vi "УОПП ПользователиZZ.vi"() -> ()   [LabVIEW 2018]
uses:
  Control 1.ctl
  <vilib>/Analysis/baseanly.llb/Mean (DBL).vi
  <vilib>/Instr/_visa.llb/VISA Configure Serial Port (Instr).vi
  <vilib>/Utility/file.llb/Write Delimited Spreadsheet (string).vi
  <vilib>/addons/control/pid/pid.llb/PID (DBL).vi
  <vilib>/NI/Modbus Library/API/Master/Modbus Master.lvclass
  <vilib>/addons/control/pid/NI_PID_pid.lvlib
  <vilib>/Analysis/NI_AALBase.lvlib
  <vilib>/Analysis/NI_AALPro.lvlib
panel:
  out "x > y?":bool
  in  "Наименование образца":string
  in  "OK Button 2":bool
  in  "OK Button":bool
  in  "Масса. г":dbl format="%#.3g"
  in  "Длина, мм.":dbl=30.0 min=8.0 max=150.0
  in  "Диаметр, мм.":dbl=30.0 min=8.0 max=100.0
  in  "клапан":u16=4000 format="%.3f"
  out "Boolean 10":bool
  out "Скорость падения давления":dbl format="%#.6g"
  out "y":dbl
  out "Вр1 2":dbl
  out "Вр2 3":dbl
  out "травление":bool
  out "травление3":bool
  out "травление 2":bool
  in  "error out":errorcluster
  out "Вр2":bool
  out "Boolean 9":bool
  out "Вр1":bool
  out "Boolean 7":bool
  out "Boolean 6":bool
  out "Boolean 5":bool
  out "Boolean 4":bool
  out "Boolean 3":bool
  in  "Штангель":dbl format="%#.3g"
  out "Время":dbl[](array[numeric])
  out "Пересчет":dbl[](array[numeric])
  out "Atm":dbl[](array[numeric])
  out "Vip":dbl[](array[numeric])
  out "Вип":dbl
  out "Вип 3":dbl
  out "Вип 2":dbl
  out "Вип 4":dbl
  out "Вип 5":dbl
  out "pori 4":dbl
  out "pori 2":dbl
  out "Tab Control 2":enum32{"Page 1", "Page 2", "Page 3"}(tab)=enum."Page 3"
  out "Проницаемость. мД":dbl
  out "Пористость. %":dbl format="%#.6f"
  out "P_пл.МПа":dbl format="%#.2g"
  out "P пл. МПа":dbl format="%#.2g"
  out "P гор. МПа":dbl format="%#.2g"
  out "Нижний":bool
  out "Верхний":bool
  out "K11":bool
  out "K10":bool
  out "K9":bool=TRUE
  out "K8":bool
  out "K7":bool
  out "K6":bool
  out "K5":bool
  out "K4":bool
  out "K3":bool
  out "K2":bool
  out "K1":bool
  out "Плотность образца.\n г/см3":dbl format="%#.3g"
  out "Объем скелета . см3":dbl format="%#.3g"
  out "Плотность зерен г/см3":dbl format="%#.3g"
  out "Плотность зерен г/см3":dbl
  out "Скорость":dbl format="%#.3g"
  out "Температура":dbl format="%#.3f"
  out "Пласт1":dbl format="%#.3g"
  out "Пласт2":dbl format="%#.3g"
  out "Ошибки":i32=1 format="%.3f"
  out "дельта":dbl format="%#.3g"
  in  "Регулятор\n давления":dbl min=0.0 max=1.5 format="%#.3f"
  in  "Пластовое давл.":dbl=1.5 min=0.0 max=1.5 format="%#.3g"
  out "Рпласт.":dbl(graph)
  in  "Min":dbl=0.05 format="%#.3g"
  in  "Max":dbl=0.62 format="%#.3g"
  out "Y":dbl format="%#.3g"
  out "X":dbl format="%#.3g"
  out "Pатм. МПа":dbl format="%#.3f"
  out "Пористость. %":dbl format="%#.3f"
  out "P2/P1":dbl[](array[numeric])
  out "Pпластовое":dbl format="%#.5f"
  out "Проницаемость. мД":dbl format="%#.3g"
  out "P_пластовое МПа":dbl format="%#.6f"
  out "Объем скелета . см3":dbl format="%#.3g"
  out "Плотность образца.\n г/см3":dbl format="%#.3g"
  out "0,17":dbl
  out "0,2":dbl
  out "0,25":dbl
  out "0,15":dbl
  out "D 0,4":dbl
  in  "stop 3":bool=TRUE
  in  "Клапана":bool[](array[boolean])=[FALSE, FALSE, FALSE, FALSE, FALSE, FALSE, FALSE, FALSE, TRUE, FALSE, FALSE, FALSE, FALSE]
  out "String 2":T1="     К1         К2         К3         К4          К5          К6         К7         К8         К9        К10         К11 "
  in  "Продувка":bool
  out "n 1":dbl
  out "n 2":dbl
  out "n 3":dbl
  out "n 4":dbl
  out "n":dbl
  out "D2":dbl
  out "D3":dbl
  out "D4":dbl
  out "D1":dbl
  out "Q":dbl
  out "Q 2":dbl
  out "Q 3":dbl
  out "Q 4":dbl
  out "Q 3.2":dbl
  out "pori 3":dbl
  out "XY Graph 2":cluster{dbl[], dbl[]}[](graph)
  out "секунды 2":dbl format="%#.3g"
  out "0,38":dbl
  out "Low level pronic":dbl
  out "pori 1":dbl
  out "T0.5":u32
  out "T1":u32
  out "T2":u32
  out "appended array":dbl[](array[numeric])
  out "sum":dbl
  out "Прол":dbl
  in  "Сохранение данных":bool
  in  "Укажите место для сохранения файла":path
  in  "Boolean 8":bool
  out "Table Control":string[][](table)
  in  "Save Button":bool=TRUE
  in  "stop 2":bool
  in  "Режимы":u16(ring)=1 items=["Проницаемость", "Пористость"]
  in  "Старт":bool
  out "Темп":dbl format="%0.2f"
  in  "Up Button":bool
  in  "Down Button":bool
  out "Р горное, МПа":sgl format="%#.2f"
  in  "Мультипликатор":dbl(slide) min=0.0 max=70.0 scale=0.0..70.0
  out "Атмосферное":dbl(knob) scale=0.0..1.0
  in  "код":string
  in  "Калибровка":bool
  in  "РД-1 1,0 МПА":dbl min=0.0 max=100.0 step=0.01 format="%#.3f"
  in  "РД-2 1,0 МПА":dbl=0.078 min=0.0 max=100.0 step=0.01 format="%#.2f"
  in  "PID gains":T2={"proportional gain (Kc)"=50.0, "integral time (Ti, min)"=4.0, "derivative time (Td, min)"=0.0} {"derivative time (Td, min)" format="%.3f"; "integral time (Ti, min)" format="%.3f"; "proportional gain (Kc)" format="%.3f"}
  out "output":dbl=4000.0 format="%.2f"
  in  "dt (s)":dbl=5.0 format="%.3f"
  in  "baud rate (9600)":u32=9600
  in  "ms to wait":u32=40
  out "Press":dbl format="%5.6f"
  out "Boolean 2":bool=TRUE
  out "Numeric 2":i32
  out "Numeric":i32
  # "Введите параметры образца"
  # "К 30"
  # "К 100"
  # "N2"
  # "Регулятор\n давления"
  # "He"
  # "Емкость 1"
  # "Емкость 2"
  # "Емкость 3"
  # "Емкость 4"
  # "Емкость 5"
  # "Емкость 6"
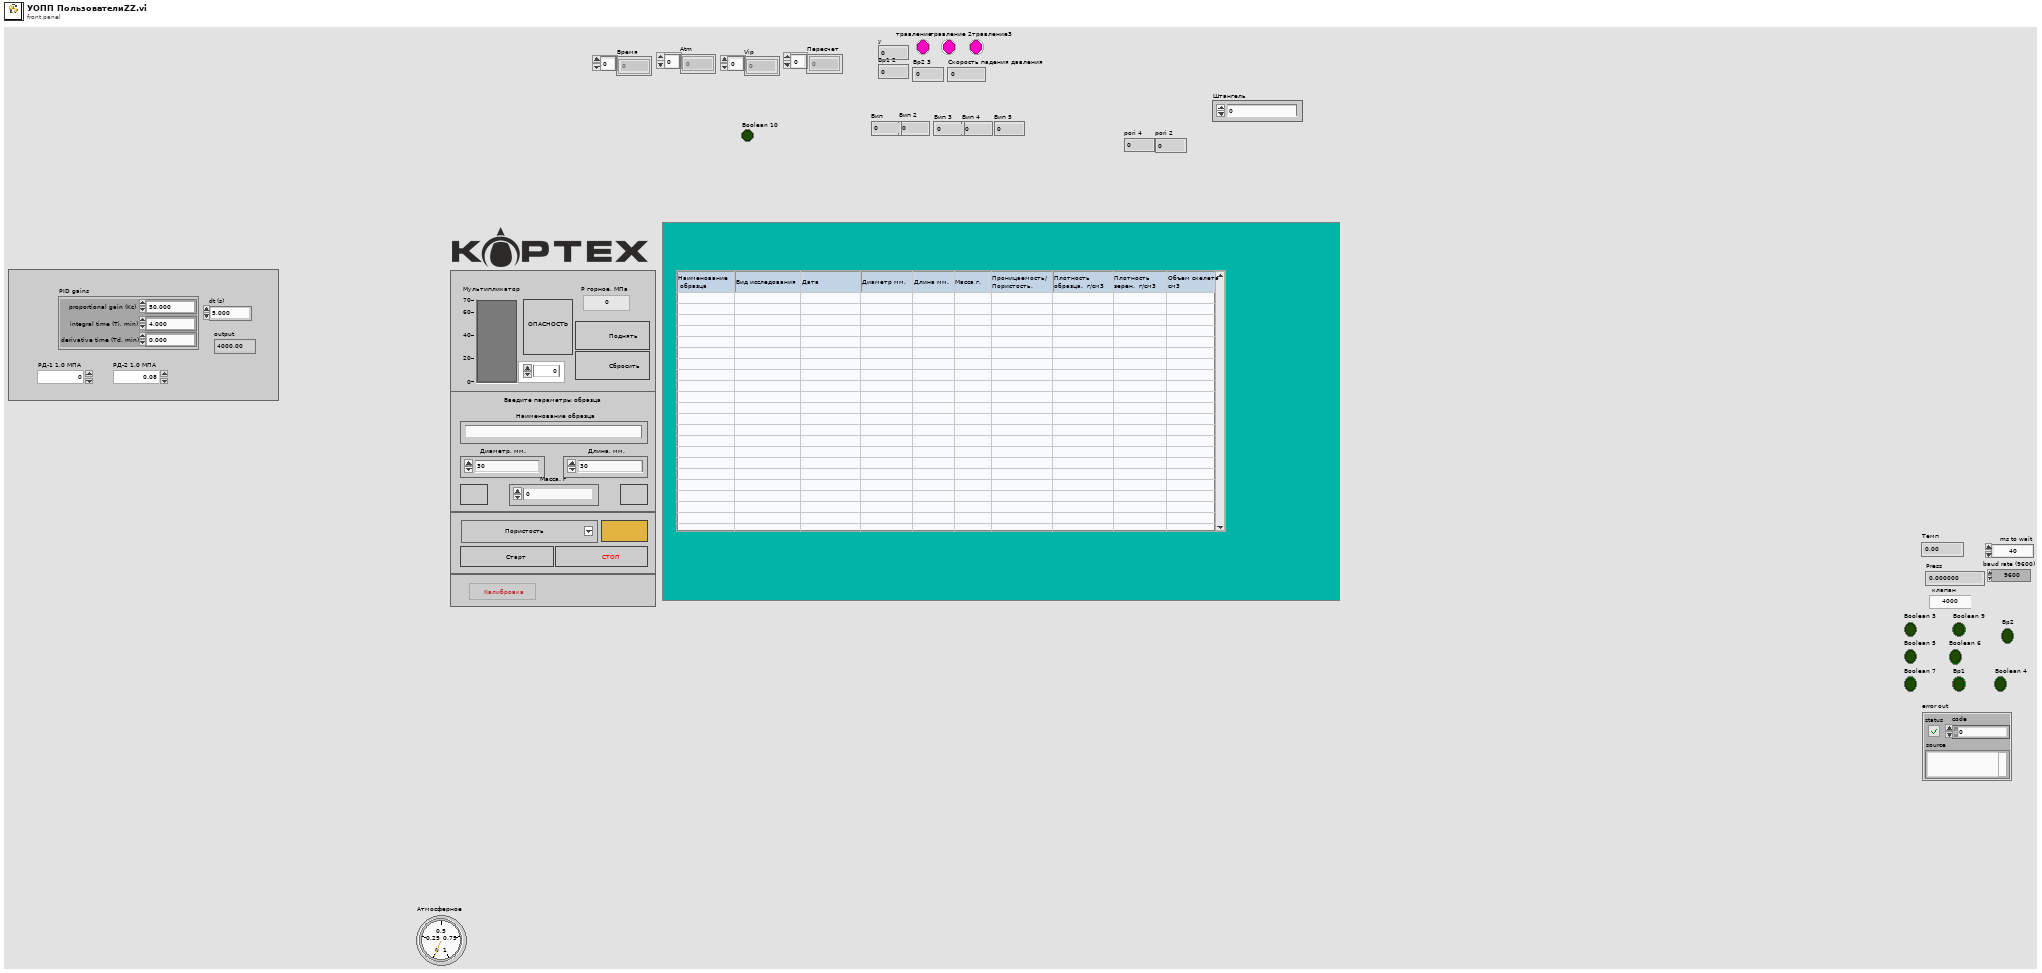
[diagram p1: front panel]
types:
  T1 = typedef "Control 1.ctl" = string
  T2 = cluster{"proportional gain (Kc)":dbl, "integral time (Ti, min)":dbl, "derivative time (Td, min)":dbl}
  T3 = enum8{"Enabled", "Disabled", "Disabled and Grayed Out"}
  T4 = typedef "Датчики.ctl" = cluster{"Клапана":T5, "Концевики":T6, "Рег.давления":T7, "Давления":cluster{"Р горное":sgl, "Р пластовое":sgl, "Р атм.":sgl, "Температура":sgl, "Р_пластовое":sgl}}
  T5 = typedef "Клапана.ctl" = cluster{"Ka-1":bool, "Ka-2":bool, "Ka-3":bool, "Ka-4":bool, "Ka-5":bool, "Ka-6":bool, "Ka-7":bool, "Ka-8":bool, "Ka-9":bool, "Ka-10":bool, "Ka-11":bool, "Ka-12":bool, "Ka-13":bool}
  T6 = typedef "Концевики.ctl" = cluster{"Di-1":bool, "Di-2":bool}
  T7 = typedef "Регуляторы.ctl" = cluster{"Рег.№1":u16, "Рег.№2":u16, "Рег.№3":u16}
  T8 = cluster{"Время":dbl[], "Best Polynomial Fit":dbl[]}
  T9 = cluster{"Время":dbl[], "Best Polynomial Fit":dbl[]}[]
  T10 = enum32{"invalid app kind", "Development System", "Run Time System", "Student Edition", "Embedded LabVIEW", "Evaluation", "Custom"}
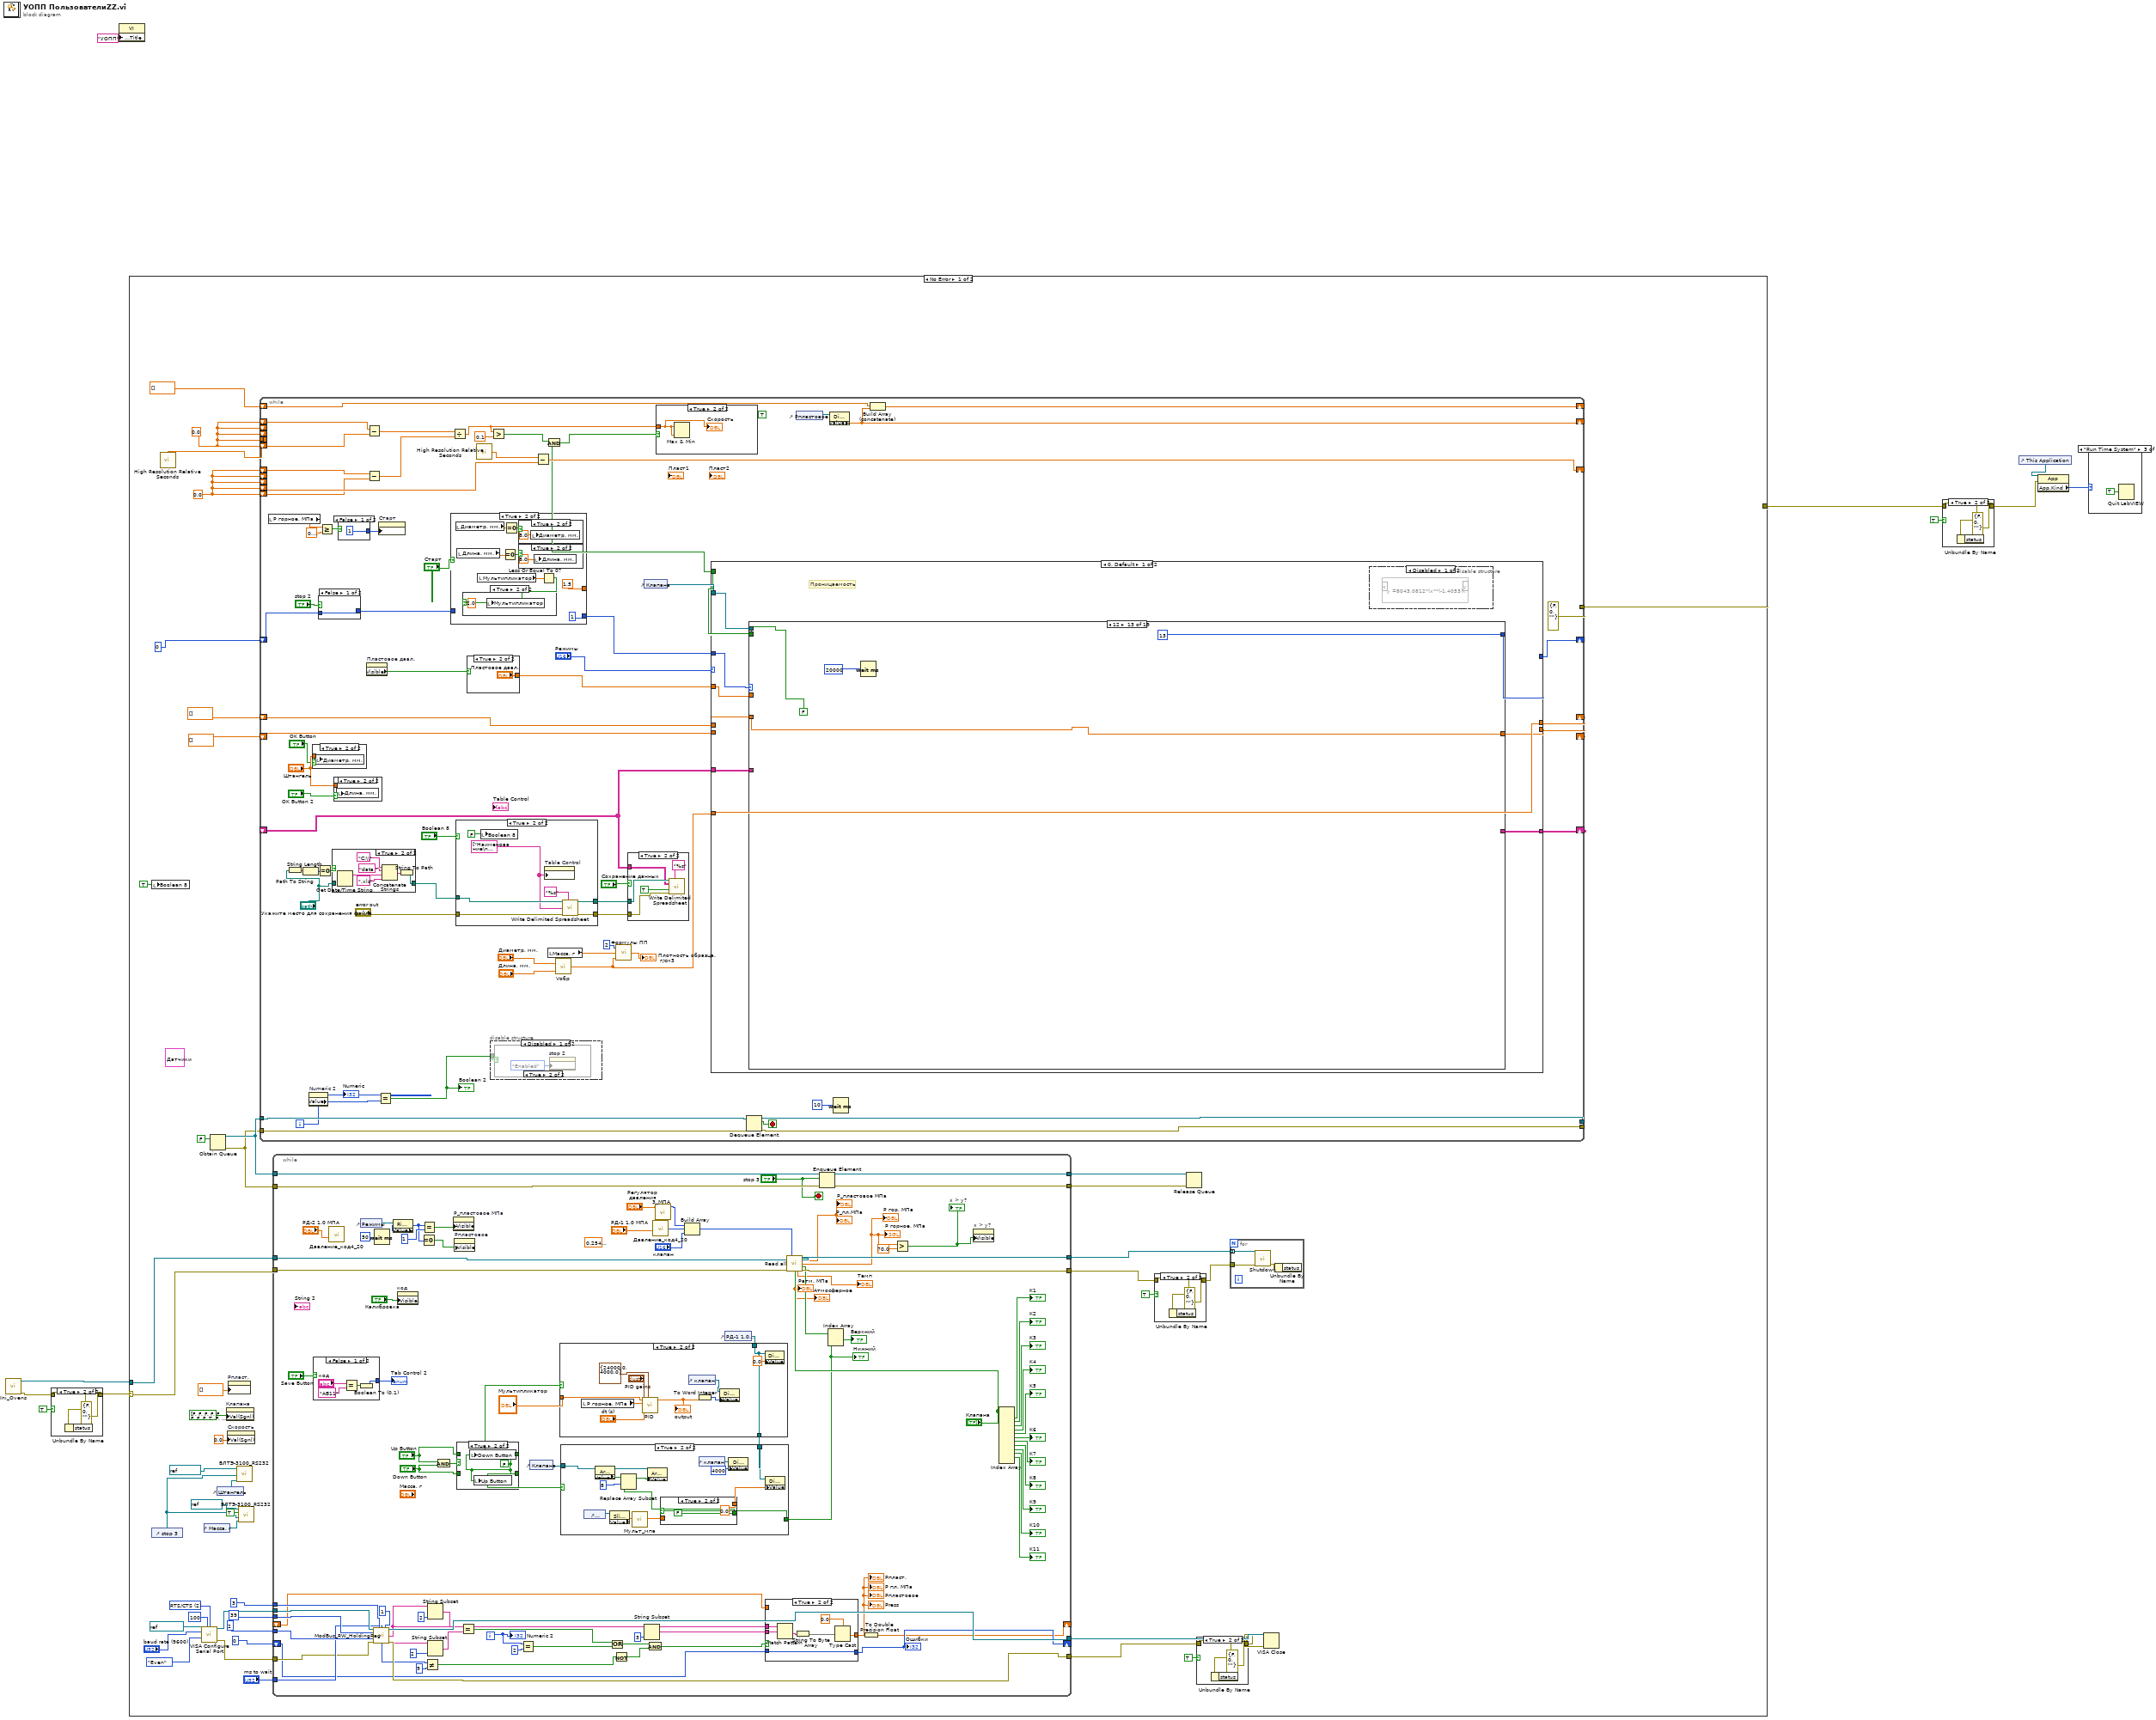
[diagram p0: block diagram]
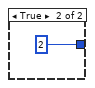
[diagram p8: hidden frame]
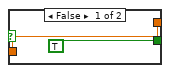
[diagram p11: hidden frame]
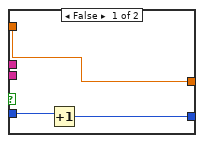
[diagram p12: hidden frame]
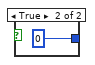
[diagram p15: hidden frame]
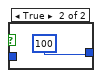
[diagram p18: hidden frame]
diagram:
  n1 = call "Ini_Ovens.vi"() -> ("error out"=w5:errorcluster, "Овны"=w10:refnum<class "Modbus Master.lvclass">[])  [unwired: 10 in]
  n2 = case shown="True" TRUE {
    tunnel: [w11 errorcluster {"status"=FALSE, "code"=0, "source"=""} ("error IO")] -> w6
    tunnel: w5 -> [w11 w12]
    frame False {
    }
    frame True {
      n3 = Unbundle By Name(w12) -> ()  [unwired: 1 out]
    }
  }
  n4 = property class="VI"("Front Panel Window:Title"="УОПП") -> ()  [unwired: 2 in, 2 out]
  n5 = case shown="No Error" w6 {
    selector: w6 -> [w51 _]
    tunnel: w10 -> [w50 _]
    tunnel: [w49 _] -> w3
    frame No Error {
      w36 = u16 2 items=["None", "XON/XOFF", "RTS/CTS", "XON/XOFF & RTS/CTS", "DTR/DSR", "XON/XOFF & DTR/DSR"] ("flow control (0:none)")
      w43 = 0.0
      w48 = 0.0
      (unwired) T4 {"Клапана"={"Ka-1"=FALSE, "Ka-2"=FALSE, "Ka-3"=FALSE, "Ka-4"=FALSE, "Ka-5"=FALSE, "Ka-6"=FALSE, "Ka-7"=FALSE, "Ka-8"=FALSE, "Ka-9"=FALSE, "Ka-10"=FALSE, "Ka-11"=FALSE, "Ka-12"=FALSE, "Ka-13"=FALSE}, "Концевики"={"Di-1"=FALSE, "Di-2"=FALSE}, "Рег.давления"={"Рег.№1"=0, "Рег.№2"=0, "Рег.№3"=0}, "Давления"={"Р горное"=0.0, "Р пластовое"=0.0, "Р атм."=0.0, "Температура"=0.0, "Р_пластовое"=0.0}} ("Датчики")
      n6 = local write "Boolean 8"(TRUE ("Boolean 8")) -> ()
      n7 = control-ref of="stop 3"() -> (w14:refnum<vi>)
      n8 = call <vilib>:"High Resolution Relative Seconds.vi"() -> ("relative seconds"=w47:dbl)
      n9 = call-poly "VISA Configure Serial Port"("VISA resource name"=refnum<visa-resource-name> "COM10" ("VISA Refnum in"), "timeout (10sec)"=u32 100, "baud rate (9600)"="baud rate (9600)", "parity (0:none)"=enum16{"None", "Odd", "Even", "Mark", "Space"}."Even", "flow control (0:none)"=w36) -> ("VISA resource name out"=w33:refnum<visa-resource-name>, "error out"=w31:errorcluster)  [unwired: 9 in]
      n10 = control-ref of="Масса. г"() -> (w19:refnum<vi>)
      n11 = Obtain Queue(element data type=FALSE) -> (queue out=w57:refnum<queue>, error out=w44:errorcluster)  [unwired: 4 in, 1 out]
      n12 = control-ref of="Штангель"() -> (w15:refnum<vi>)
      n13 = property on="Клапана" class="Arr (strict)"("Val(Sgnl)"=bool[] [FALSE, FALSE, FALSE, FALSE, FALSE, FALSE, FALSE, FALSE, TRUE, FALSE, FALSE, FALSE, FALSE] ("Value (Signaling)")) -> ()  [unwired: 2 in, 2 out]
      n14 = property on="Скорость" class="DigNum (strict)"("Val(Sgnl)"=0.0 ("Value (Signaling)")) -> ()  [unwired: 2 in, 2 out]
      n15 = property on="Рпласт." class="WFChart (strict)"("History Data"=sgl[] []) -> ()  [unwired: 2 in, 2 out]
      n16 = call "ВЛТЭ-3100_RS232.vi"("Balance 2"=w15, "Stop 2"=w14, "VISA resource name"=refnum<visa-resource-name> "COM3") -> ()  [unwired: 2 in]
      n17 = call "ВЛТЭ-3100_RS232.vi"("Balance 2"=w19, "Stop 2"=w14, "0,001"=TRUE, "VISA resource name"=refnum<visa-resource-name> "COM5") -> ()  [unwired: 1 in]
      n18 = while {
        tunnel: w57 -> [w268]
        tunnel: w44 -> [w266]
        tunnel: [w265] -> _
        tunnel: [w264] -> _
        tunnel: [errorcluster {"status"=FALSE, "code"=0, "source"=""} ("error in (no error)")] -> w49
        shift-right: [w245] -> _
        shift-left: w48 -> [w261]
        shift-left: w48 -> [_]
        shift-left: w48 -> [_]
        shift-left: w48 -> [_]
        shift-left: w48 -> [w260]
        shift-right: [w257] -> _
        shift-left: w43 -> [w256]
        shift-left: w43 -> [_]
        shift-left: w43 -> [_]
        shift-left: w43 -> [_]
        shift-left: w43 -> [w255]
        tunnel: w47 -> [w258]
        shift-right: [w247] -> _
        shift-left: 0 -> [w223]
        shift-right: [w237] -> _
        shift-left: dbl[] [] -> [w238]
        shift-right: [w234] -> _
        shift-left: dbl[] [] -> [w233]
        shift-right: [w231] -> _
        shift-left: dbl[] [] -> [w232]
        shift-right: [w207] -> _
        shift-left: _ -> [w206]
        i -> [w241]
        stop <- w267 stop-if-true
        (unwired) TRUE
        n19 = local read "Р горное, МПа"() -> (w221:sgl)
        n20 = Path To String(path="Укажите место для сохранения файла") -> (string=w214:string)
        n21 = String Length(string=w214) -> (length=w215:i32)
        n22 = property on="Numeric 2" class="DigNum (strict)"() -> ("Value"=w243:i32)  [unwired: 2 in, 2 out]
        n23 = case shown="True" "OK Button" {
          tunnel: "Штангель" -> [_ w295]
          frame False {
          }
          frame True {
            n24 = local write "Диаметр, мм."(w295) -> ()
          }
        }
        n25 = Equal To 0?(x=w215) -> (x = 0?=w213:bool)
        n26 = case shown="False" "stop 2" {
          tunnel: w223 -> [w292 _]
          tunnel: [w292 100] -> w222
          frame False {
          }
          frame True {
          }
        }
        n27 = Greater Or Equal?(x=w221, y=sgl 0.9) -> (x >= y?=w218:bool)
        n28 = case shown="True" w213 {
          tunnel: "Укажите место для сохранения файла" -> [w276 _]
          tunnel: [w276 w277] -> w211
          frame False {
          }
          frame True {
            n29 = Get Date/Time String() -> (date string=w282:string)  [unwired: 3 in, 1 out]
            n30 = Concatenate Strings("C:\\" ("string"), "data " ("default name"), w282, ".xls" ("string")) -> (w278:string)
            n31 = String To Path(string=w278) -> (path=w277:path)
          }
        }
        n32 = case shown="True" "OK Button 2" {
          tunnel: "Штангель" -> [_ w294]
          frame False {
          }
          frame True {
            n33 = local write "Длина, мм."(w294) -> ()
          }
        }
        n34 = case shown="False" w218 {
          tunnel: [1 0] -> w219
          frame False {
          }
          frame True {
          }
        }
        n35 = Subtract(x=w261, y=w260) -> (x-y=w254:dbl)
        n36 = Subtract(x=w256, y=w255) -> (x-y=w253:dbl)
        n37 = property on="Пластовое давл." class="DigNum (strict)"() -> ("Visible"=w235:bool)  [unwired: 2 in, 2 out]
        n38 = Equal?(x=w241, y=w243) -> (x = y?=w242:bool)
        "Boolean 2" <- w242
        n39 = property on="Старт" class="Bool (strict)"("DisabledEnum"=w219) -> ()  [unwired: 2 in, 2 out]
        n40 = case shown="True" "Старт" {
          tunnel: [w1028 1] -> w246
          tunnel: [0.0 ("Начальное давл.") 1.5 ("Начальное давл.")] -> _
          tunnel: w222 -> [w1028 _]
          frame False {
          }
          frame True {
            n41 = local read "Диаметр, мм."() -> (w1033:dbl)
            n42 = local read "Длина, мм."() -> (w1031:dbl)
            n43 = local read "Мультипликатор"() -> (w1034:dbl)
            n44 = Equal To 0?(x=w1031) -> (x = 0?=w1030:bool)
            n45 = Equal To 0?(x=w1033) -> (x = 0?=w1032:bool)
            n46 = case shown="True" w1032 {
              frame False {
              }
              frame True {
                n47 = local write "Диаметр, мм."(8.0 ("Диаметр. мм.")) -> ()
              }
            }
            n48 = case shown="True" w1030 {
              frame False {
              }
              frame True {
                n49 = local write "Длина, мм."(8.0 ("Диаметр. мм.")) -> ()
              }
            }
            n50 = Less Or Equal To 0?(x=w1034) -> (x <= 0?=w1035:bool)
            n51 = case shown="True" w1035 {
              frame False {
              }
              frame True {
                n52 = local write "Мультипликатор"(2.0 ("Мультиплексор.МПА")) -> ()
              }
            }
          }
        }
        n53 = Divide(x=w254, y=w253) -> (x/y=w252:dbl)
        n54 = case shown="True" "Boolean 8" {
          tunnel: [w284 w290] -> w209
          tunnel: [w283 w289] -> w208
          tunnel: w211 -> [w284 w286]
          tunnel: "error out" -> [w283 w288]
          frame False {
          }
          frame True {
            w285 = string[] ["Наименование\n образца", "Вид исследования", "Дата", "Диаметр мм.", "Длина мм.", "Масса г.", "Проницаемость/\nПористость.", "Плотность\nобразца.  г/см3", "Плотность\nзерен.  г/см3", "Объем скелета\nсм3 "] ("Array 2")
            n55 = local write "Boolean 8"(FALSE ("Boolean 8")) -> ()
            n56 = property on="Table Control" class="Tbl (strict)"("Column Headers[]"=w285) -> ()  [unwired: 2 in, 2 out]
            n57 = call-poly <vilib>:"Write Delimited Spreadsheet.vi"("file path (dialog if empty)"=w286, "format (%s)"="%s", "1D data"=w285, "error in (no error)"=w288) -> ("new file path (Not A Path if cancelled)"=w290:path, "error out"=w289:errorcluster)  [unwired: 10 in]
          }
        }
        n58 = case shown="True" w235 {
          tunnel: [1.5 ("Пластовое давл.") "Пластовое давл."] -> w239
          frame False {
          }
          frame True {
          }
        }
        n59 = call <vilib>:"High Resolution Relative Seconds.vi"() -> ("relative seconds"=w259:dbl)
        n60 = disable-structure shown="Disabled" {
          disable-tunnel: w242 -> [w296 _]
          frame Disabled {
            n61 = case shown="True" w296 {
              frame False {
              }
              frame True {
                n62 = property on="stop 2" class="Bool (strict)"("DisabledEnum"=T3."Enabled" ("Disabled")) -> ()  [unwired: 2 in, 2 out]
              }
            }
          }
          frame Enabled {
          }
        }
        n63 = Greater?(x=w252, y=0.1) -> (0:w250:bool)
        n64 = Subtract(x=w259, y=w258) -> (x-y=w257:dbl)
        n65 = local read "Масса. г"() -> (w204:dbl)
        n66 = call "Vобр.vi"("Длина, мм."="Длина, мм.", "Диаметр. мм."="Диаметр, мм.") -> ("Объем образца см3"=w203:dbl)
        n67 = call "Формулы ПП.vi"("PerB"=w203, "PerA"=w204, "mode"=2) -> ("Exid"=→"Плотность образца.\n г/см3":dbl)
        n68 = case shown="True" "Сохранение данных" {
          tunnel: w209 -> [_ w271]
          tunnel: w208 -> [_ w270]
          tunnel: w206 -> [_ w269]
          frame False {
          }
          frame True {
            n69 = call-poly <vilib>:"Write Delimited Spreadsheet.vi"("file path (dialog if empty)"=w271, "format (%s)"="%s" ("format (%.3f)"), "2D data"=w269, "append to file? (new file:F)"=TRUE, "error in (no error)"=w270) -> ()  [unwired: 9 in, 2 out]
          }
        }
        n70 = control-ref of="Клапана"() -> (w248:refnum<vi>)
        n71 = case shown="0, Default" "Режимы" {
          tunnel: w248 -> [w308 w737]
          tunnel: [w302 w734] -> w247
          tunnel: w246 -> [w306 w735]
          tunnel: [w307 w733] -> w244
          tunnel: w239 -> [w309 w736]
          tunnel: [w305 w732] -> w234
          tunnel: w233 -> [w305 w731]
          tunnel: w232 -> [w304 w730]
          tunnel: [w303 w730] -> w231
          tunnel: w203 -> [_ w729]
          tunnel: [w300 w728] -> w207
          tunnel: w206 -> [w301 w727]
          frame 0, Default {
            # "Проницаемость"
            n72 = case shown="12" w306 {
              selector: w306 -> [w314 _ _ _ _ _ _ _ _ _ _ _ _ _ _ _ _ _ _]
              tunnel: [w314 2 w333 4 5 6 7 w416 9 10 11 12 13 14 0 51 52 7 w691] -> w302
              tunnel: w308 -> [_ w325 _ w357 _ w378 _ _ _ _ _ w618 _ w634 _ w647 _ w681 w694]
              tunnel: [FALSE FALSE FALSE FALSE FALSE FALSE FALSE FALSE FALSE FALSE FALSE TRUE FALSE FALSE FALSE FALSE FALSE FALSE FALSE] -> w307
              tunnel: w309 -> [_ w321 _ _ _ _ _ _ _ _ _ _ _ _ _ _ _ _ _]
              tunnel: w304 -> [w311 w319 w336 w355 w366 w375 w386 _ w567 w590 w603 w614 w625 w631 w644 w655 w658 w683 w692]
              tunnel: [w310 w318 w335 w354 w365 w374 w385 w408 w566 dbl[] [] w602 w614 w625 w631 w644 w655 w658 w683 w692] -> w303
              tunnel: [_ _ _ _ _ _ _ _ _ _ w600 _ _ _ _ _ _ _ _] -> w300
              tunnel: w301 -> [_ _ _ _ _ _ _ _ _ _ w598 _ _ _ _ _ _ _ _]
              frame 0, Default {
                n73 = local read "Темп"() -> (w312:dbl)
                n74 = Build Array (concatenate)(w311, w312) -> (w310:dbl[])
              }
              frame 1 {
                w315 = 0.0 ("Пористость. %")
                w316 = TRUE ("new element/subarray")
                n75 = property on="Регулятор\n давления" class="DigNum (strict)"("Value"=w321) -> ()  [unwired: 2 in, 2 out]
                n76 = property class="Arr (strict)"(reference=w325) -> (reference out=w328:refnum<vi>, error out=w327:errorcluster, "Value"=w329:bool[])  [unwired: 1 in]
                n77 = Replace Array Subset(array=w329, new element #1=w316, index #1=0 ("index"), new element #2=w316, index #2=9 ("index"), new element #3=w316, index #3=4, new element #4=w316, index #4=2 ("index"), new element #5=w316, index #5=5 ("index")) -> (w326:bool[])
                n78 = property class="Arr (strict)"(reference=w328, error in=w327, "Value"=w326) -> ()  [unwired: 2 out]
                n79 = local read "Темп"() -> (w320:dbl)
                n80 = Build Array (concatenate)(w319, w320) -> (w318:dbl[])
                n81 = local write "Пористость. %"(w315) -> ()
                n82 = local write "Плотность образца.\n г/см3"(w315) -> ()
                n83 = local write "Объем скелета . см3"(w315) -> ()
                n84 = local write "Плотность зерен г/см3"(w315) -> ()
                n85 = local write "Проницаемость. мД"(w315) -> ()
              }
              frame 2 {
                n86 = call <vilib>:"High Resolution Relative Seconds.vi"() -> ("relative seconds"=w334:dbl)
                n87 = while {
                  tunnel: w334 -> [w347]
                  tunnel: [3] -> w333
                  stop <- w340 stop-if-true
                  n88 = local read "Max"() -> (w339:dbl)
                  n89 = call <vilib>:"High Resolution Relative Seconds.vi"() -> ("relative seconds"=w348:dbl)
                  n90 = Subtract(x=w348, y=w347) -> (x-y=w346:dbl)
                  n91 = property on="Pпластовое" class="DigNum (strict)"() -> ("Value"=w349:dbl)  [unwired: 2 in, 2 out]
                  n92 = Greater Or Equal?(x=w346, y=120.0) -> (x >= y?=w342:bool)
                  n93 = Greater?(x=w349, y=w339) -> (0:w343:bool)
                  n94 = local read "stop 2"() -> (w341:bool)
                  n95 = Compound Arithmetic op=OR(w343, w342, w341) -> (w340:bool)
                }
                n96 = local read "Темп"() -> (w337:dbl)
                n97 = Build Array (concatenate)(w336, w337) -> (w335:dbl[])
              }
              frame 3 {
                w352 = FALSE ("new element/subarray")
                (unwired) 1.5 ("VPPL-3L")
                n98 = property on="Регулятор\n давления" class="DigNum (strict)"("Value"=0.0 ("VPPL-3L")) -> ()  [unwired: 2 in, 2 out]
                n99 = property class="Arr (strict)"(reference=w357) -> (reference out=w360:refnum<vi>, error out=w361:errorcluster, "Value"=w359:bool[])  [unwired: 1 in]
                n100 = property on="Регулятор\n давления" class="DigNum (strict)"("Value"=0.0 ("VPPL-3L")) -> ()  [unwired: 2 in, 2 out]
                n101 = Replace Array Subset(array=w359, new element #1=w352, index #1=0 ("index"), new element #2=w352, index #2=9 ("index")) -> (w362:bool[])
                n102 = property class="Arr (strict)"(reference=w360, error in=w361, "Value"=w362) -> ()  [unwired: 2 out]
                n103 = local read "Темп"() -> (w356:dbl)
                n104 = Build Array (concatenate)(w355, w356) -> (w354:dbl[])
              }
              frame 4 {
                n105 = Wait (ms)(milliseconds to wait=u32 15000) -> ()  [unwired: 1 out]
                n106 = local read "Темп"() -> (w367:dbl)
                n107 = Build Array (concatenate)(w366, w367) -> (w365:dbl[])
              }
              frame 5 {
                w371 = TRUE ("Boolean 3")
                n108 = local write "травление"(w371) -> ()
                n109 = local write "травление 2"(w371) -> ()
                n110 = local write "травление3"(w371) -> ()
                n111 = local write "Boolean 9"(w371) -> ()
                n112 = property class="Arr (strict)"(reference=w378) -> (reference out=w372:refnum<vi>, error out=w382:errorcluster, "Value"=w383:bool[])  [unwired: 1 in]
                n113 = Replace Array Subset(array=w383, new element=TRUE ("new element/subarray"), index=3) -> (w381:bool[])
                n114 = property class="Arr (strict)"(reference=w372, error in=w382, "Value"=w381) -> ()  [unwired: 2 out]
                n115 = local read "Темп"() -> (w376:dbl)
                n116 = Build Array (concatenate)(w375, w376) -> (w374:dbl[])
                "Boolean 3" <- w371
                "Boolean 4" <- w371
                "Boolean 5" <- w371
                "Boolean 6" <- w371
                "Boolean 7" <- w371
              }
              frame 6 {
                n117 = call <vilib>:"High Resolution Relative Seconds.vi"() -> ("relative seconds"=w388:dbl)
                n118 = while {
                  tunnel: [w401] -> _
                  shift-right: [w397] -> w385
                  shift-left: w386 -> [w398]
                  tunnel: w388 -> [w395]
                  stop <- w392 stop-if-true
                  (unwired) 1600000 ("x")
                  n119 = call <vilib>:"High Resolution Relative Seconds.vi"() -> ("relative seconds"=w396:dbl)
                  n120 = property on="Max" class="DigNum (strict)"() -> ("Visible"=w400:bool)  [unwired: 2 in, 2 out]
                  n121 = Subtract(x=w396, y=w395) -> (x-y=w394:dbl)
                  n122 = case shown="True" w400 {
                    tunnel: [0.7 "Max"] -> w401
                    frame False {
                    }
                    frame True {
                    }
                  }
                  n123 = property on="Pпластовое" class="DigNum (strict)"() -> ("Value"=w403:dbl)  [unwired: 2 in, 2 out]
                  n124 = Less Or Equal?(x=w403, y=w401) -> (x <= y?=w391:bool)
                  n125 = local read "stop 2"() -> (w389:bool)
                  n126 = Greater Or Equal?(x=w394, y=120.0) -> (x >= y?=w390:bool)
                  n127 = Wait Until Next ms Multiple(millisecond multiple=u32 10) -> ()  [unwired: 1 out]
                  n128 = Compound Arithmetic op=OR(w391, w390, w389) -> (w392:bool)
                  n129 = local read "Темп"() -> (w399:dbl)
                  n130 = Build Array (concatenate)(w398, w399) -> (w397:dbl[])
                }
              }
              frame 7 {
                w406 = TRUE ("Вр1")
                n131 = local write "Boolean 9"(w406) -> ()
                n132 = local write "Вр1"(w406) -> ()
                n133 = local write "Вр2"(w406) -> ()
                n134 = call <vilib>:"High Resolution Relative Seconds.vi"() -> ("relative seconds"=w413:dbl)
                n135 = while {
                  tunnel: [w446] -> w414 mode=indexing
                  tunnel: [w448] -> w409 mode=indexing
                  tunnel: w413 -> [w470]
                  tunnel: [w469] -> _
                  tunnel: [w422] -> w412 mode=indexing
                  shift-right: [w460] -> w408
                  shift-left: dbl[] [] -> [w467]
                  tunnel: [w461] -> w410 mode=indexing
                  stop <- w464 stop-if-true
                  (unwired) 2147483647 ("y")
                  n136 = property on="Min" class="DigNum (strict)"() -> ("Visible"=w468:bool)  [unwired: 2 in, 2 out]
                  n137 = local read "травление"() -> (w449:bool)
                  n138 = local read "травление 2"() -> (w450:bool)
                  n139 = local read "травление3"() -> (w451:bool)
                  n140 = case shown="True" w468 {
                    tunnel: [0.15 "Min"] -> w469
                    frame False {
                    }
                    frame True {
                    }
                  }
                  n141 = call <vilib>:"High Resolution Relative Seconds.vi"() -> ("relative seconds"=w471:dbl)
                  n142 = property on="Pпластовое" class="DigNum (strict)"() -> ("Value"=w448:dbl)  [unwired: 2 in, 2 out]
                  n143 = Subtract(x=w471, y=w470) -> (x-y=w446:dbl)
                  n144 = property on="Pатм. МПа" class="DigNum (strict)"() -> ("Value"=w461:dbl)  [unwired: 2 in, 2 out]
                  n145 = local read "Вр2"() -> (w452:bool)
                  n146 = local read "stop 2"() -> (w465:bool)
                  n147 = Greater Or Equal?(x=w446, y=20.0) -> (x >= y?=w453:bool)
                  n148 = local read "Вр1"() -> (w455:bool)
                  n149 = Greater Or Equal To 0?(x=w446) -> (x >= 0?=w456:bool)
                  n150 = And(x=w453, y=w452) -> (x .and. y?=w447:bool)
                  n151 = case shown="True" w447 {
                    selector: w447 -> [w477 _]
                    tunnel: [w477 w491] -> w438
                    tunnel: w451 -> [_ w480]
                    tunnel: w450 -> [_ w484]
                    tunnel: w449 -> [_ w486]
                    tunnel: w448 -> [_ w488]
                    frame False {
                    }
                    frame True {
                      n152 = local read "Вр1 2"() -> (w489:dbl)
                      n153 = Subtract(x=w488, y=w489) -> (x-y=w493:dbl)
                      n154 = Divide(x=w493, y=10.0) -> (x/y=w481:dbl)
                      "Скорость падения давления" <- w481
                      n155 = call "Больше И.vi"("Чек"=w480, "Граница"=0.0001 ("y"), "Значение"=w481) -> ("T/F"=w478:bool)
                      n156 = call "Больше И.vi"("Чек"=w486, "Граница"=0.00083 ("y"), "Значение"=w481) -> ("T/F"=w487:bool)
                      n157 = call "Больше И.vi"("Чек"=w484, "Граница"=0.00033 ("y"), "Значение"=w481) -> ("T/F"=w482:bool)
                      n158 = Compound Arithmetic op=OR(w487, w482, w478) -> (w491:bool)
                      "Вр2 3" <- w488
                      "Вр2" <- FALSE ("Вр2")
                    }
                  }
                  "Boolean 10" <- w438
                  n159 = Less Or Equal?(x=w448, y=w469) -> (x <= y?=w463:bool)
                  n160 = call "Формула Проницаемости.vi"("Р атм.."=w461, "P пластовое"=w448) -> ("Давление по пересчету"=w422:dbl)  [unwired: 9 in]
                  n161 = And(x=w456, y=w455) -> (x .and. y?=w454:bool)
                  n162 = Greater Or Equal?(x=w446, y=600.0) -> (x >= y?=w462:bool)
                  n163 = case shown="True" w454 {
                    tunnel: w448 -> [_ w495]
                    frame False {
                    }
                    frame True {
                      "Вр1 2" <- w495
                      "Вр1" <- FALSE ("Вр1")
                    }
                  }
                  n164 = local read "Темп"() -> (w459:dbl)
                  n165 = Build Array (concatenate)(w467, w459) -> (w460:dbl[])
                  n166 = call-poly <vilib>:"Mean.vi"("X"=w460) -> ("mean"=w458:dbl)  [unwired: 1 out]
                  n167 = local read "Boolean 9"() -> (w420:bool)
                  n168 = local read "Boolean 4"() -> (w433:bool)
                  n169 = local read "Boolean 3"() -> (w435:bool)
                  n170 = local read "Boolean 5"() -> (w429:bool)
                  n171 = local read "Boolean 6"() -> (w426:bool)
                  n172 = local read "Boolean 7"() -> (w424:bool)
                  n173 = call "Больше И.vi"("Чек"=w420, "Граница"=0.38 ("y"), "Значение"=w422) -> ("T/F"=w421:bool)
                  n174 = call "Больше И.vi"("Чек"=w429, "Граница"=0.2 ("y"), "Значение"=w422) -> ("T/F"=w431:bool)
                  n175 = call "Больше И.vi"("Чек"=w433, "Граница"=0.25 ("y"), "Значение"=w422) -> ("T/F"=w434:bool)
                  n176 = call "Больше И.vi"("Чек"=w435, "Граница"=0.4 ("y"), "Значение"=w422) -> ("T/F"=w437:bool)
                  n177 = call "Больше И.vi"("Чек"=w424, "Граница"=0.15 ("y"), "Значение"=w422) -> ("T/F"=w423:bool)
                  n178 = call "Больше И.vi"("Чек"=w426, "Граница"=0.17 ("y"), "Значение"=w422) -> ("T/F"=w428:bool)
                  n179 = And(x=w421, y=w438) -> (x .and. y?=w445:bool)
                  n180 = Compound Arithmetic op=OR(w462, w463, w465, w445) -> (w464:bool)
                  n181 = case shown="True" w421 {
                    tunnel: w446 -> [_ w475]
                    tunnel: w438 -> [_ _]
                    frame False {
                    }
                    frame True {
                      n182 = local read "D 0,4"() -> (w476:dbl)
                      n183 = Subtract(x=w475, y=w476) -> (x-y=w473:dbl)
                      "0,38" <- w473
                      n184 = formula code="pro=227.074650314*dt**(-0.931628294);"("dt"=w473) -> ("pro"=→"Low level pronic":dbl)
                      "Boolean 9" <- FALSE ("Boolean 9")
                    }
                  }
                  n185 = case shown="True" w423 {
                    tunnel: w446 -> [_ w500]
                    tunnel: w461 -> [_ w506]
                    tunnel: w458 -> [_ w505]
                    tunnel: w448 -> [_ w501]
                    frame False {
                    }
                    frame True {
                      n186 = local read "0,17"() -> (w499:dbl)
                      n187 = local read "n 3"() -> (w504:dbl)
                      n188 = local write "Boolean 7"(FALSE ("Boolean 3")) -> ()
                      n189 = call "VAT.vi"("Разность"=w504, "Temper"=w505, "Атмосферное"=w506, "Вип"=w501) -> ("n"=→"n 4":dbl, "раз"=w497:dbl)
                      n190 = Subtract(x=w500, y=w499) -> (x-y=w496:dbl)
                      "D4" <- w496
                      n191 = call "Qpori.vi"("Dt"=w496, "Dn"=w497) -> ("pori"=→"pori 4":dbl, "Q"=→"Q 4":dbl)  [unwired: 1 in]
                      "0,15" <- w500
                      "Вип 5" <- w501
                    }
                  }
                  n192 = case shown="True" w437 {
                    tunnel: w446 -> [_ w549]
                    tunnel: w448 -> [_ w545]
                    tunnel: w461 -> [_ w548]
                    tunnel: w458 -> [_ w547]
                    frame False {
                    }
                    frame True {
                      n193 = call "VAT.vi"("Temper"=w547, "Атмосферное"=w548, "Вип"=w545) -> ("n"=→"n":dbl)  [unwired: 1 in, 1 out]
                      n194 = local write "Boolean 3"(FALSE ("Boolean 3")) -> ()
                      "D 0,4" <- w549
                      "Вип" <- w545
                    }
                  }
                  n195 = case shown="True" w431 {
                    tunnel: w446 -> [_ w525]
                    tunnel: w458 -> [_ w530]
                    tunnel: w461 -> [_ w529]
                    tunnel: w448 -> [_ w526]
                    frame False {
                    }
                    frame True {
                      n196 = local read "0,25"() -> (w524:dbl)
                      n197 = local read "n 1"() -> (w528:dbl)
                      n198 = call "VAT.vi"("Разность"=w528, "Temper"=w530, "Атмосферное"=w529, "Вип"=w526) -> ("n"=→"n 2":dbl, "раз"=w522:dbl)
                      n199 = local write "Boolean 5"(FALSE ("Boolean 3")) -> ()
                      n200 = Subtract(x=w525, y=w524) -> (x-y=w521:dbl)
                      "D2" <- w521
                      n201 = call "Qpori.vi"("Dt"=w521, "Dn"=w522) -> ("pori"=→"pori 2":dbl, "Q"=→"Q 2":dbl)  [unwired: 1 in]
                      "0,2" <- w525
                      "Вип 3" <- w526
                    }
                  }
                  n202 = case shown="True" w428 {
                    tunnel: w446 -> [_ w512]
                    tunnel: w458 -> [_ w514]
                    tunnel: w461 -> [_ w518]
                    tunnel: w448 -> [_ w513]
                    frame False {
                    }
                    frame True {
                      n203 = local read "0,2"() -> (w511:dbl)
                      n204 = local read "n 2"() -> (w517:dbl)
                      n205 = call "VAT.vi"("Разность"=w517, "Temper"=w514, "Атмосферное"=w518, "Вип"=w513) -> ("n"=→"n 3":dbl, "раз"=w509:dbl)
                      n206 = local write "Boolean 6"(FALSE ("Boolean 3")) -> ()
                      n207 = Subtract(x=w512, y=w511) -> (x-y=w508:dbl)
                      "D3" <- w508
                      n208 = call "Qpori.vi"("Dt"=w508, "Dn"=w509) -> ("pori"=→"pori 3":dbl, "Q"=→"Q 3":dbl)  [unwired: 1 in]
                      "0,17" <- w512
                      "Вип 4" <- w513
                    }
                  }
                  n209 = case shown="True" w434 {
                    tunnel: w446 -> [_ w536]
                    tunnel: w458 -> [_ w542]
                    tunnel: w461 -> [_ w541]
                    tunnel: w448 -> [_ w537]
                    frame False {
                    }
                    frame True {
                      n210 = local read "D 0,4"() -> (w543:dbl)
                      n211 = local read "n"() -> (w540:dbl)
                      n212 = call "VAT.vi"("Разность"=w540, "Temper"=w542, "Атмосферное"=w541, "Вип"=w537) -> ("n"=→"n 1":dbl, "раз"=w535:dbl)
                      n213 = local write "Boolean 4"(FALSE ("Boolean 3")) -> ()
                      n214 = Subtract(x=w536, y=w543) -> (x-y=w534:dbl)
                      "D1" <- w534
                      n215 = call "Qpori.vi"("Dt"=w534, "Numeric"=0, "Dn"=w535) -> ("pori"=→"pori 1":dbl, "Q"=→"Q":dbl)
                      "0,25" <- w536
                      "Вип 2" <- w537
                    }
                  }
                  n216 = local read "Q 2"() -> (w443:dbl)
                  n217 = local read "Q 3"() -> (w442:dbl)
                  n218 = local read "Q 4"() -> (w441:dbl)
                  n219 = local read "Q"() -> (w444:dbl)
                  n220 = Build Array(w444, w443, w442, w441) -> (w440:dbl[])
                  n221 = Add Array Elements(numeric array=w440) -> (sum=w439:dbl)
                  n222 = call "QQQQQQ.vi"("Q"=w439) -> ()  [unwired: 1 out]
                }
                "Vip" <- w409
                "Atm" <- w410
                "Пересчет" <- w412
                "Время" <- w414
                n223 = case shown="False" FALSE {
                  tunnel: [8 50] -> w416
                  frame False {
                  }
                  frame True {
                  }
                }
              }
              frame 8 {
                n224 = local read "Пересчет"() -> (w565:dbl[])
                n225 = local read "Atm"() -> (w562:dbl[])
                n226 = local read "Vip"() -> (w556:dbl[])
                n227 = local read "Время"() -> (w555:dbl[])
                n228 = local read "Темп"() -> (w574:dbl)
                n229 = Array Size(array=w555) -> (size(s)=w579:i32)
                n230 = Build Array (concatenate)(w567, w574) -> (w566:dbl[])
                n231 = Decrement(x=w579) -> (x-1=w578:i32)
                n232 = Index Array(array=w555, index=w578) -> (element=→"секунды 2":dbl)
                n233 = call-poly <vilib>:"Mean.vi"("X"=w566) -> ("mean"=w573:dbl)  [unwired: 1 out]
                n234 = call <vilib>:"General Polynomial Fit.vi"("Y"=w556, "X"=w555) -> ("Best Polynomial Fit"=w554:dbl[])  [unwired: 10 in, 3 out]
                n235 = call "Диапазоны Delta.vi"("Вип"=w554, "Пересчет"=w565, "Atm"=w562, "Время"=w555, "Temper"=w573) -> ("output cluster"=w576:cluster{"Время":dbl[], dbl[]}, "appended array"=→"appended array":dbl[], "Q"=→"Q 3.2":dbl)  [unwired: 1 in, 1 out]
                n236 = Bundle("Время"=w555, "Best Polynomial Fit"=w554) -> (w563:T8)  [unwired: 1 in]
                n237 = Build Array(w563, w576) -> (→"XY Graph 2":T9)
                n238 = local read "D1"() -> (w558:dbl)
                n239 = local read "D2"() -> (w572:dbl)
                n240 = local read "D3"() -> (w571:dbl)
                n241 = local read "D4"() -> (w570:dbl)
                n242 = local read "Q"() -> (w557:dbl)
                n243 = Build Array(w558, w572, w571, w570) -> (w560:dbl[])
                n244 = call "Scaling and Mapping"("Signals"=w557) -> ("Scaled Signals"=→"Прол":dynamicdata)  [unwired: 9 in, 1 out]
                n245 = Add Array Elements(numeric array=w560) -> (sum=w553:dbl)
                "sum" <- w553
                n246 = call "Scaling and Mapping4"("Signals"=w553) -> ()  [unwired: 9 in, 2 out]
                n247 = call "Scaling and Mapping3"("Signals"=w553) -> ()  [unwired: 9 in, 2 out]
              }
              frame 9 {
                n248 = Wait (ms)(milliseconds to wait=u32 5000) -> ()  [unwired: 1 out]
                n249 = local read "Темп"() -> (w591:dbl)
                n250 = Build Array (concatenate)(w590, w591) -> (w582:dbl[])
                n251 = call-poly <vilib>:"Mean.vi"("X"=w582) -> ("mean"=w588:dbl)  [unwired: 1 out]
                "Температура" <- w588
                n252 = call "температура азот.vi"("Температура"=w588) -> ("вязкость"=w587:dbl)  [unwired: 10 in]
                n253 = local read "Boolean 10"() -> (w580:bool)
                n254 = call "температура азот.vi"("Температура"=25.0) -> ("вязкость"=w586:dbl)  [unwired: 10 in]
                n255 = Divide(x=w587, y=w586) -> (x/y=w585:dbl)
                n256 = case shown="False" w580 {
                  tunnel: [w595 w596] -> w581
                  frame False {
                    n257 = local read "Прол"() -> (w595:dbl)
                  }
                  frame True {
                    n258 = local read "Low level pronic"() -> (w596:dbl)
                  }
                }
                n259 = Multiply(x=w585, y=w581) -> (x*y=→"Проницаемость. мД":dbl)
              }
              frame 10 {
                n260 = local read "Проницаемость. мД"() -> (w601:dbl)
                n261 = local read "Наименование образца"() -> (w597:string)
                n262 = local read "Масса. г"() -> (w605:dbl)
                n263 = local read "Диаметр, мм."() -> (w607:dbl)
                n264 = local read "Длина, мм."() -> (w608:dbl)
                n265 = call "Datatxt.vi"("Наименование образца"=w597, "string"="Проницаемость", "Масса"=w605, "длина"=w608, "Диаметр"=w607, "Пористость"=w601) -> ("appended array"=w599:string[])  [unwired: 5 in]
                n266 = Build Array (concatenate)(w598, w599) -> (w600:string[][])
                n267 = local read "Темп"() -> (w604:dbl)
                n268 = property on="Регулятор\n давления" class="DigNum (strict)"("Value"=0.0 ("VPPL-3L")) -> ()  [unwired: 2 in, 2 out]
                n269 = Build Array (concatenate)(w603, w604) -> (w602:dbl[])
              }
              frame 11 {
                w613 = FALSE ("new element/subarray")
                n270 = property class="Arr (strict)"(reference=w618) -> (reference out=w622:refnum<vi>, error out=w621:errorcluster, "Value"=w623:bool[])  [unwired: 1 in]
                n271 = Replace Array Subset(array=w623, new element #1=TRUE ("new element/subarray"), index #1=1 ("index"), new element #2=w613, index #2=4 ("index"), new element #3=w613, index #3=5 ("index")) -> (w620:bool[])
                n272 = property class="Arr (strict)"(reference=w622, error in=w621, "Value"=w620) -> ()  [unwired: 2 out]
              }
              frame 12 {
                n273 = Wait (ms)(milliseconds to wait=u32 20000) -> ()  [unwired: 1 out]
              }
              frame 13 {
                w630 = FALSE ("new element/subarray")
                n274 = property class="Arr (strict)"(reference=w634) -> (reference out=w638:refnum<vi>, error out=w639:errorcluster, "Value"=w637:bool[])  [unwired: 1 in]
                n275 = Replace Array Subset(array=w637, new element #1=w630, index #1=1 ("index"), new element #2=w630, index #2=3 ("index"), new element #3=w630, index #3=2 ("index")) -> (w640:bool[])
                n276 = property class="Arr (strict)"(reference=w638, error in=w639, "Value"=w640) -> ()  [unwired: 2 out]
              }
              frame 14 {
                n277 = local read "Проницаемость. мД"() -> (→"Проницаемость. мД":dbl)
                n278 = property on="Клапана" class="Arr (strict)"("DisabledEnum"=T3."Enabled" ("Disabled")) -> ()  [unwired: 2 in, 2 out]
                n279 = Wait (ms)(milliseconds to wait=u32 2000) -> ()  [unwired: 1 out]
              }
              frame 50 {
                n280 = property class="Arr (strict)"(reference=w647) -> (reference out=w651:refnum<vi>, error out=w652:errorcluster, "Value"=w650:bool[])  [unwired: 1 in]
                n281 = Replace Array Subset(array=w650, new element=TRUE ("new element/subarray"), index=1) -> (w653:bool[])
                n282 = property class="Arr (strict)"(reference=w651, error in=w652, "Value"=w653) -> ()  [unwired: 2 out]
              }
              frame 51 {
                n283 = call <vilib>:"High Resolution Relative Seconds.vi"() -> ("relative seconds"=w660:dbl)
                n284 = while {
                  tunnel: w660 -> [w671]
                  stop <- w666 stop-if-true
                  n285 = local read "травление 2"() -> (w661:bool)
                  n286 = local read "травление"() -> (w663:bool)
                  n287 = call <vilib>:"High Resolution Relative Seconds.vi"() -> ("relative seconds"=w672:dbl)
                  n288 = case shown="True" w661 {
                    selector: w661 -> [w674 _]
                    tunnel: [0.19 ("y") w677] -> w665
                    tunnel: w663 -> [_ w676]
                    frame False {
                      "травление3" <- w674
                    }
                    frame True {
                      n289 = case shown="False" w676 {
                        selector: w676 -> [w678 _]
                        tunnel: [0.21 ("y") 0.33 ("y")] -> w677
                        frame False {
                          "травление 2" <- w678
                        }
                        frame True {
                        }
                      }
                    }
                  }
                  "y" <- w665
                  n290 = Subtract(x=w672, y=w671) -> (x-y=w670:dbl)
                  n291 = property on="Pпластовое" class="DigNum (strict)"() -> ("Value"=w673:dbl)  [unwired: 2 in, 2 out]
                  n292 = Greater Or Equal?(x=w670, y=120.0) -> (x >= y?=w668:bool)
                  n293 = local read "stop 2"() -> (w667:bool)
                  n294 = Less?(x=w673, y=w665) -> (x < y?=w664:bool)
                  n295 = Compound Arithmetic op=OR(w664, w668, w667) -> (w666:bool)
                  n296 = Not(x=w664) -> (.not. x?=→"травление":bool)
                }
              }
              frame 52 {
                n297 = property class="Arr (strict)"(reference=w681) -> (reference out=w688:refnum<vi>, error out=w689:errorcluster, "Value"=w687:bool[])  [unwired: 1 in]
                n298 = Replace Array Subset(array=w687, new element=FALSE ("new element/subarray"), index=1) -> (w690:bool[])
                n299 = property class="Arr (strict)"(reference=w688, error in=w689, "Value"=w690) -> ()  [unwired: 2 out]
              }
              frame 100 {
                n300 = flat-sequence {
                  tunnel: w694 -> [w709]
                  tunnel: [w697] -> w695
                  tunnel: w695 -> [w726]
                  tunnel: [0] -> w691
                  frame #0 {
                    w698 = TRUE
                    w704 = FALSE
                    n301 = property class="Arr (strict)"(reference=w709) -> (reference out=w711:refnum<vi>, error out=w712:errorcluster, "Value"=w710:bool[])  [unwired: 1 in]
                    n302 = Replace Array Subset(array=w710, new element #1=w704, index #1=0 ("index"), new element #2=w704, index #2=1 ("index"), new element #3=w704, index #3=9 ("index"), new element #4=w704, index #4=10 ("index"), new element #5=w698, index #5=2 ("index"), new element #6=w698, index #6=3 ("index"), new element #7=w698, index #7=4 ("index"), new element #8=w698, index #8=5 ("index"), new element #9=w698, index #9=6 ("index")) -> (w713:bool[])
                    n303 = property class="Arr (strict)"(reference=w711, error in=w712, "Value"=w713) -> (reference out=w697:refnum<vi>)  [unwired: 1 out]
                    n304 = Wait (ms)(milliseconds to wait=u32 20000) -> ()  [unwired: 1 out]
                  }
                  frame #1 {
                    w716 = FALSE
                    n305 = property class="Arr (strict)"(reference=w726) -> (reference out=w724:refnum<vi>, error out=w723:errorcluster, "Value"=w725:bool[])  [unwired: 1 in]
                    n306 = Replace Array Subset(array=w725, new element #1=w716, index #1=2 ("index"), new element #2=w716, index #2=3 ("index"), new element #3=w716, index #3=4 ("index"), new element #4=w716, index #4=5 ("index"), new element #5=w716, index #5=6 ("index")) -> (w722:bool[])
                    n307 = Wait (ms)(milliseconds to wait=u32 5000) -> ()  [unwired: 1 out]
                    n308 = property class="Arr (strict)"(reference=w724, error in=w723, "Value"=w722) -> ()  [unwired: 2 out]
                  }
                }
              }
            }
            n309 = disable-structure shown="Disabled" {
              frame Disabled {
                n310 = formula code="y =8043.0812*(x**(-1.4053));"() -> ()  [unwired: 1 in, 1 out]
              }
              frame Enabled {
              }
            }
          }
          frame 1 {
            # "Пористость"
            n311 = case shown="20" w735 {
              selector: w735 -> [w740 _ _ _ _ _ _ _ _ _ _ _ _ _ _ _ _ _ _ _ _ _ _ _ _]
              tunnel: [w740 w743 3 4 w775 6 7 8 9 10 11 12 w864 14 15 16 17 18 19 20 21 22 23 w969 w992] -> w734
              tunnel: w737 -> [_ w746 _ w765 _ w794 _ w808 _ w824 _ w841 _ w882 _ _ w903 _ _ w936 _ w953 _ _ w996]
              tunnel: [FALSE FALSE FALSE FALSE FALSE TRUE TRUE FALSE FALSE FALSE FALSE FALSE FALSE FALSE FALSE FALSE TRUE FALSE FALSE FALSE FALSE FALSE FALSE FALSE FALSE] -> w733
              tunnel: w736 -> [_ _ _ _ _ _ _ _ _ _ _ _ w863 _ _ _ _ _ _ _ _ _ _ _ _]
              tunnel: [w738 w744 w759 w763 w777 w791 w802 w805 w816 w821 w833 w836 w861 w879 w893 w897 w900 w917 w927 w933 w945 w948 w964 w971 w995] -> w732
              tunnel: w731 -> [w738 w744 w759 w763 w777 w791 w802 w805 w816 w821 w833 w837 w861 w879 w893 w897 w900 w917 w928 w933 w945 w948 w964 w971 w995]
              tunnel: w729 -> [_ _ _ _ _ _ _ _ _ _ _ _ _ _ _ _ _ _ w919 _ _ _ _ _ _]
              tunnel: [_ _ _ _ _ _ _ _ _ _ _ _ _ _ _ _ _ _ _ _ _ _ _ w967 _] -> w728
              tunnel: w727 -> [_ _ _ _ _ _ _ _ _ _ _ _ _ _ _ _ _ _ _ _ _ _ _ w966 _]
              frame 0, Default {
              }
              frame 1 {
                w741 = 0.0 ("Пористость. %")
                n312 = disable-structure shown="Disabled" {
                  frame Disabled {
                    n313 = property on="Клапана" class="Arr (strict)"("DisabledEnum"=T3."Disabled and Grayed Out" ("Disabled")) -> ()  [unwired: 2 in, 2 out]
                  }
                  frame Enabled {
                  }
                }
                n314 = case shown="False" "Продувка" {
                  tunnel: w746 -> [w750 _]
                  tunnel: [2 11] -> w743
                  frame False {
                    n315 = property class="Arr (strict)"(reference=w750) -> (reference out=w753:refnum<vi>, error out=w752:errorcluster, "Value"=w754:bool[])  [unwired: 1 in]
                    n316 = Replace Array Subset(array=w754, new element=TRUE ("new element/subarray"), index=2) -> (w751:bool[])
                    n317 = property class="Arr (strict)"(reference=w753, error in=w752, "Value"=w751) -> ()  [unwired: 2 out]
                  }
                  frame True {
                  }
                }
                n318 = local write "Пористость. %"(w741) -> ()
                n319 = local write "Плотность образца.\n г/см3"(w741) -> ()
                n320 = local write "Объем скелета . см3"(w741) -> ()
                n321 = local write "Плотность зерен г/см3"(w741) -> ()
                n322 = local write "Проницаемость. мД"(w741) -> ()
              }
              frame 2 {
                w757 = 0.0 ("Пористость. %")
                n323 = local write "Пористость. %"(w757) -> ()
                n324 = local write "Плотность образца.\n г/см3"(w757) -> ()
                n325 = local write "Объем скелета . см3"(w757) -> ()
                n326 = local write "Плотность зерен г/см3"(w757) -> ()
                n327 = Wait (ms)(milliseconds to wait=u32 4000) -> ()  [unwired: 1 out]
                n328 = local write "Проницаемость. мД"(0.0 ("Проницаемость. мД")) -> ()
              }
              frame 3 {
                w770 = TRUE ("new element/subarray")
                n329 = property class="Arr (strict)"(reference=w765) -> (reference out=w773:refnum<vi>, error out=w772:errorcluster, "Value"=w774:bool[])  [unwired: 1 in]
                n330 = Replace Array Subset(array=w774, new element #1=w770, index #1=0 ("index"), new element #2=w770, index #2=10 ("index"), new element #3=w770, index #3=1 ("index")) -> (w771:bool[])
                n331 = property class="Arr (strict)"(reference=w773, error in=w772, "Value"=w771) -> ()  [unwired: 2 out]
              }
              frame 4 {
                n332 = call <vilib>:"High Resolution Relative Seconds.vi"() -> ("relative seconds"=w776:dbl)
                n333 = while {
                  tunnel: [5] -> w775
                  tunnel: w776 -> [w788]
                  stop <- w779 stop-if-true
                  n334 = call <vilib>:"High Resolution Relative Seconds.vi"() -> ("relative seconds"=w787:dbl)
                  n335 = Subtract(x=w787, y=w788) -> (x-y=w786:dbl)
                  n336 = Equal?(x=w786, y=25.0) -> (x = y?=w781:bool)
                  n337 = property on="P_пластовое МПа" class="DigNum (strict)"() -> ("Value"=w784:dbl)  [unwired: 2 in, 2 out]
                  n338 = Greater Or Equal?(x=w784, y=0.5) -> (x >= y?=w782:bool)
                  n339 = local read "stop 2"() -> (w780:bool)
                  n340 = Compound Arithmetic op=OR(w782, w781, w780) -> (w779:bool)
                }
              }
              frame 5 {
                w792 = FALSE ("new element/subarray")
                n341 = property class="Arr (strict)"(reference=w794) -> (reference out=w798:refnum<vi>, error out=w797:errorcluster, "Value"=w799:bool[])  [unwired: 1 in]
                n342 = Replace Array Subset(array=w799, new element #1=w792, index #1=0 ("index"), new element #2=w792, index #2=10 ("index")) -> (w796:bool[])
                n343 = property class="Arr (strict)"(reference=w798, error in=w797, "Value"=w796) -> ()  [unwired: 2 out]
              }
              frame 6 {
                n344 = Wait (ms)(milliseconds to wait=u32 10000) -> ()  [unwired: 1 out]
              }
              frame 7 {
                n345 = property class="Arr (strict)"(reference=w808) -> (reference out=w812:refnum<vi>, error out=w813:errorcluster, "Value"=w811:bool[])  [unwired: 1 in]
                n346 = Replace Array Subset(array=w811, new element=TRUE ("new element/subarray"), index=3) -> (w814:bool[])
                n347 = property class="Arr (strict)"(reference=w812, error in=w813, "Value"=w814) -> ()  [unwired: 2 out]
              }
              frame 8 {
                n348 = Wait (ms)(milliseconds to wait=u32 4000) -> ()  [unwired: 1 out]
              }
              frame 9 {
                w819 = FALSE ("new element/subarray")
                n349 = property class="Arr (strict)"(reference=w824) -> (reference out=w830:refnum<vi>, error out=w829:errorcluster, "Value"=w831:bool[])  [unwired: 1 in]
                n350 = Replace Array Subset(array=w831, new element #1=w819, index #1=3 ("index"), new element #2=w819, index #2=2 ("index"), new element #3=w819, index #3=1 ("index")) -> (w828:bool[])
                n351 = property class="Arr (strict)"(reference=w830, error in=w829, "Value"=w828) -> ()  [unwired: 2 out]
                n352 = property on="Клапана" class="Arr (strict)"("DisabledEnum"=T3."Enabled" ("Disabled")) -> ()  [unwired: 2 in, 2 out]
              }
              frame 10 {
                n353 = Wait (ms)(milliseconds to wait=u32 3000) -> ()  [unwired: 1 out]
              }
              frame 11 {
                w844 = TRUE ("new element/subarray")
                n354 = property class="Arr (strict)"(reference=w841) -> (reference out=w849:refnum<vi>, error out=w850:errorcluster, "Value"=w848:bool[])  [unwired: 1 in]
                n355 = Replace Array Subset(array=w848, new element #1=w844, index #1=0 ("index"), new element #2=w844, index #2=10 ("index"), new element #3=w844, index #3=1 ("index")) -> (w851:bool[])
                n356 = Array Size(array=w837) -> (size(s)=w840:i32)
                n357 = property class="Arr (strict)"(reference=w849, error in=w850, "Value"=w851) -> ()  [unwired: 2 out]
                n358 = Equal?(x=w840, y=3) -> (x = y?=w838:bool)
                n359 = property on="Клапана" class="Arr (strict)"("DisabledEnum"=T3."Disabled and Grayed Out" ("Disabled")) -> ()  [unwired: 2 in, 2 out]
                n360 = case shown="True" w838 {
                  tunnel: [w853 dbl[] []] -> w836
                  tunnel: w837 -> [w853 _]
                  frame False {
                  }
                  frame True {
                  }
                }
              }
              frame 12 {
                n361 = property on="Регулятор\n давления" class="DigNum (strict)"("Value"=w863) -> ()  [unwired: 2 in, 2 out]
                n362 = call <vilib>:"High Resolution Relative Seconds.vi"() -> ("relative seconds"=w860:dbl)
                n363 = while {
                  tunnel: [13] -> w864
                  tunnel: w860 -> [w874]
                  stop <- w865 stop-if-true
                  n364 = call <vilib>:"High Resolution Relative Seconds.vi"() -> ("relative seconds"=w873:dbl)
                  n365 = Subtract(x=w873, y=w874) -> (x-y=w872:dbl)
                  n366 = Equal?(x=w872, y=25.0) -> (x = y?=w867:bool)
                  n367 = property on="P_пластовое МПа" class="DigNum (strict)"() -> ("Value"=w870:dbl)  [unwired: 2 in, 2 out]
                  n368 = local read "stop 2"() -> (w866:bool)
                  n369 = Greater Or Equal?(x=w870, y=1.0) -> (x >= y?=w868:bool)
                  n370 = Compound Arithmetic op=OR(w868, w867, w866) -> (w865:bool)
                }
                n371 = Wait (ms)(milliseconds to wait=u32 10000) -> (millisecond timer value=w856:u32)
                n372 = Wait (ms)(milliseconds to wait=u32 0) -> (millisecond timer value=w855:u32)
                n373 = Subtract(x=w856, y=w855) -> (x-y=→"T0.5":u32)
              }
              frame 13 {
                w878 = FALSE ("new element/subarray")
                n374 = property on="Регулятор\n давления" class="DigNum (strict)"("Value"=0.0 ("VPPL-3L")) -> ()  [unwired: 2 in, 2 out]
                n375 = property class="Arr (strict)"(reference=w882) -> (reference out=w884:refnum<vi>, error out=w885:errorcluster, "Value"=w883:bool[])  [unwired: 1 in]
                n376 = Replace Array Subset(array=w883, new element #1=w878, index #1=0 ("index"), new element #2=w878, index #2=10 ("index")) -> (w886:bool[])
                n377 = property class="Arr (strict)"(reference=w884, error in=w885, "Value"=w886) -> ()  [unwired: 2 out]
              }
              frame 14 {
                n378 = Wait (ms)(milliseconds to wait=u32 0) -> (millisecond timer value=w888:u32)
                n379 = Wait (ms)(milliseconds to wait=u32 2000) -> (millisecond timer value=w889:u32)
                n380 = Subtract(x=w889, y=w888) -> (x-y=→"T1":u32)
              }
              frame 15 {
                n381 = property on="P_пластовое МПа" class="DigNum (strict)"() -> ("Value"=w896:dbl)  [unwired: 2 in, 2 out]
                n382 = local write "Пласт1"(w896) -> ()
              }
              frame 16 {
                n383 = property class="Arr (strict)"(reference=w903) -> (reference out=w905:refnum<vi>, error out=w906:errorcluster, "Value"=w904:bool[])  [unwired: 1 in]
                n384 = Replace Array Subset(array=w904, new element=TRUE ("new element/subarray"), index=2) -> (w907:bool[])
                n385 = property class="Arr (strict)"(reference=w905, error in=w906, "Value"=w907) -> ()  [unwired: 2 out]
              }
              frame 17 {
                n386 = Wait (ms)(milliseconds to wait=u32 5000) -> (millisecond timer value=w911:u32)
                n387 = Wait (ms)(milliseconds to wait=u32 0) -> (millisecond timer value=w910:u32)
                n388 = Subtract(x=w911, y=w910) -> (x-y=→"T2":u32)
              }
              frame 18 {
                n389 = local read "Пласт1"() -> (w932:dbl)
                n390 = property on="P_пластовое МПа" class="DigNum (strict)"() -> ("Value"=w931:dbl)  [unwired: 2 in, 2 out]
                n391 = local write "Пласт2"(w931) -> ()
                n392 = Divide(x=w931, y=w932) -> (x/y=w926:dbl)
                "X" <- w926
                n393 = Build Array (concatenate)(w928, w926) -> (w927:dbl[])
                "P2/P1" <- w927
                n394 = Subtract(x=w932, y=w931) -> (x-y=→"дельта":dbl)
                n395 = call-poly <vilib>:"Mean.vi"("X"=w927) -> ("mean"=w918:dbl)  [unwired: 1 out]
                n396 = call "Формула пористости.vi"("Объем образца"=w919, "V пористости P2/P1"=w918) -> ("Пористость %"=→"Пористость. %":dbl, "объем скелета"=w921:dbl, "Y"=→"Y":dbl)
                "Объем скелета . см3" <- w921
                n397 = local read "Масса. г"() -> (w924:dbl)
                n398 = Divide(x=w924, y=w921) -> (x/y=→"Плотность зерен г/см3":dbl)
              }
              frame 19 {
                n399 = property class="Arr (strict)"(reference=w936) -> (reference out=w939:refnum<vi>, error out=w938:errorcluster, "Value"=w940:bool[])  [unwired: 1 in]
                n400 = Replace Array Subset(array=w940, new element=TRUE ("new element/subarray"), index=3) -> (w937:bool[])
                n401 = property class="Arr (strict)"(reference=w939, error in=w938, "Value"=w937) -> ()  [unwired: 2 out]
              }
              frame 20 {
                n402 = Wait (ms)(milliseconds to wait=u32 5000) -> ()  [unwired: 1 out]
              }
              frame 21 {
                w949 = FALSE ("new element/subarray")
                n403 = property class="Arr (strict)"(reference=w953) -> (reference out=w956:refnum<vi>, error out=w957:errorcluster, "Value"=w955:bool[])  [unwired: 1 in]
                n404 = property on="Регулятор\n давления" class="DigNum (strict)"("Value"=0.0 ("VPPL-3L")) -> ()  [unwired: 2 in, 2 out]
                n405 = Replace Array Subset(array=w955, new element #1=w949, index #1=2 ("index"), new element #2=w949, index #2=3 ("index"), new element #3=w949, index #3=10 ("index"), new element #4=w949, index #4=1 ("index")) -> (w958:bool[])
                n406 = property on="Клапана" class="Arr (strict)"("DisabledEnum"=T3."Enabled" ("Disabled")) -> ()  [unwired: 2 in, 2 out]
                n407 = property class="Arr (strict)"(reference=w956, error in=w957, "Value"=w958) -> ()  [unwired: 2 out]
              }
              frame 22 {
                n408 = Wait (ms)(milliseconds to wait=u32 2000) -> ()  [unwired: 1 out]
              }
              frame 23 {
                n409 = Array Size(array=w971) -> (size(s)=w970:i32)
                n410 = Equal?(x=w970, y=3) -> (x = y?=w972:bool)
                n411 = case shown="True" w972 {
                  tunnel: [11 0] -> w969
                  tunnel: w971 -> [w975 _]
                  tunnel: [w975 dbl[] []] -> _
                  tunnel: [w974 w979] -> w967
                  tunnel: w966 -> [w974 w978]
                  frame False {
                  }
                  frame True {
                    n412 = local read "Плотность образца.\n г/см3"() -> (w983:dbl)
                    "Плотность образца.\n г/см3" <- w983
                    n413 = local read "Плотность зерен г/см3"() -> (w982:dbl)
                    "Плотность зерен г/см3" <- w982
                    n414 = local read "Пористость. %"() -> (w989:dbl)
                    n415 = local read "Масса. г"() -> (w986:dbl)
                    n416 = local read "Диаметр, мм."() -> (w988:dbl)
                    n417 = local read "Длина, мм."() -> (w987:dbl)
                    n418 = local read "Объем скелета . см3"() -> (w981:dbl)
                    "Объем скелета . см3" <- w981
                    n419 = local read "Пористость. %"() -> (→"Пористость. %":dbl)
                    n420 = call "Datatxt.vi"("Объем скелета . см3"=w981, "Плотность зерен г/см3"=w982, "Наименование образца"="Наименование образца", "Плотность образца.\n г/см3"=w983, "string"="Пористость", "Масса"=w986, "длина"=w987, "Диаметр"=w988, "Пористость"=w989) -> ("appended array"=w980:string[])  [unwired: 2 in]
                    n421 = Build Array (concatenate)(w978, w980) -> (w979:string[][])
                  }
                }
              }
              frame 100 {
                n422 = flat-sequence {
                  tunnel: w996 -> [w1010]
                  tunnel: [w998] -> w994
                  tunnel: w994 -> [w1027]
                  tunnel: [0] -> w992
                  frame #0 {
                    w999 = TRUE
                    w1005 = FALSE
                    n423 = property class="Arr (strict)"(reference=w1010) -> (reference out=w1012:refnum<vi>, error out=w1013:errorcluster, "Value"=w1011:bool[])  [unwired: 1 in]
                    n424 = Replace Array Subset(array=w1011, new element #1=w1005, index #1=0 ("index"), new element #2=w1005, index #2=1 ("index"), new element #3=w1005, index #3=9 ("index"), new element #4=w1005, index #4=10 ("index"), new element #5=w999, index #5=2 ("index"), new element #6=w999, index #6=3 ("index"), new element #7=w999, index #7=4 ("index"), new element #8=w999, index #8=5 ("index"), new element #9=w999, index #9=6 ("index")) -> (w1014:bool[])
                    n425 = property class="Arr (strict)"(reference=w1012, error in=w1013, "Value"=w1014) -> (reference out=w998:refnum<vi>)  [unwired: 1 out]
                    n426 = Wait (ms)(milliseconds to wait=u32 20000) -> ()  [unwired: 1 out]
                  }
                  frame #1 {
                    w1017 = FALSE
                    n427 = property class="Arr (strict)"(reference=w1027) -> (reference out=w1025:refnum<vi>, error out=w1024:errorcluster, "Value"=w1026:bool[])  [unwired: 1 in]
                    n428 = Replace Array Subset(array=w1026, new element #1=w1017, index #1=2 ("index"), new element #2=w1017, index #2=3 ("index"), new element #3=w1017, index #3=4 ("index"), new element #4=w1017, index #4=5 ("index"), new element #5=w1017, index #5=6 ("index")) -> (w1023:bool[])
                    n429 = Wait (ms)(milliseconds to wait=u32 5000) -> ()  [unwired: 1 out]
                    n430 = property class="Arr (strict)"(reference=w1025, error in=w1024, "Value"=w1023) -> ()  [unwired: 2 out]
                  }
                }
              }
            }
          }
        }
        n431 = And(x=w250, y=w244) -> (x .and. y?=w249:bool)
        n432 = case shown="True" w249 {
          tunnel: w252 -> [_ w1041]
          frame False {
          }
          frame True {
            n433 = Max & Min(x=w1041, y=w1041) -> ()  [unwired: 2 out]
            "Скорость" <- w1041
          }
        }
        n434 = Dequeue Element(queue=w268, error in (no error)=w266) -> (queue out=w264:refnum<queue>, element=w267:bool, error out=w265:errorcluster)  [unwired: 1 in, 1 out]
        n435 = control-ref of="Pпластовое"() -> (w236:refnum<vi>)
        n436 = property class="DigNum (strict)"(reference=w236) -> ("Value"=w245:dbl)  [unwired: 1 in, 2 out]
        n437 = Wait (ms)(milliseconds to wait=u32 10 ("millisecond multiple")) -> ()  [unwired: 1 out]
        n438 = Build Array (concatenate)(w238, w245) -> (w237:dbl[])
        "Numeric" <- w241
      }
      n439 = while {
        tunnel: w57 -> [w153]
        tunnel: [w152] -> w56
        tunnel: [w151] -> w55
        tunnel: w44 -> [w150]
        tunnel: w51 -> [w140]
        tunnel: w50 -> [w149]
        tunnel: [w148] -> w25
        tunnel: [w147] -> w54
        tunnel: u8 3 ("Func") -> [w139]
        tunnel: w33 -> [w138]
        tunnel: u16 39 ("StartAdr") -> [w137]
        tunnel: u16 2 ("StartAdr") -> [w136]
        tunnel: "ms to wait" -> [w135]
        tunnel: [w133] -> w38
        tunnel: [w132] -> w22
        tunnel: w31 -> [w131]
        shift-right: [w73] -> _
        shift-left: _ -> [w111]
        shift-right: [w109] -> _
        shift-left: 0 -> [w110]
        i -> [w114]
        stop <- "stop 3" stop-if-true
        (unwired) sgl 0.255 ("Давления.Р пластовое")
        n440 = case shown="False" "Save Button" {
          tunnel: [w155 i16 2 ("0, 1")] -> w71
          frame False {
            n441 = Equal?(x="код", y="AB11") -> (x = y?=w158:bool)
            n442 = Boolean To (0,1)(Boolean=w158) -> (0, 1=w155:i16)
          }
          frame True {
          }
        }
        "Tab Control 2" <- w71
        n443 = call "Давление_код4_20.vi"("Уставка давления"="РД-2 1,0 МПА") -> ()  [unwired: 10 in, 1 out]
        n444 = control-ref of="Режимы"() -> (w107:refnum<vi>)
        n445 = call "ModBus_RW_HoldingReg.vi"("VISA Refnum in"=w138, "Func"=w139, "milliseconds to wait"=w135, "Num/ of sensor"=1, "StartAdr"=w137, "Qanity"=w136, "error in (no error)"=w131) -> ("VISA Refnum out"=w133:refnum<visa-resource-name>, "read buffer"=w127:string, "return count"=w122:u32, "String w/o CRC"=w125:string, "error out"=w132:errorcluster)  [unwired: 3 in, 1 out]
        n446 = Wait (ms)(milliseconds to wait=u32 50) -> ()  [unwired: 1 out]
        n447 = property class="Ring (strict)"(reference=w107) -> ("Value"=w84:u16)  [unwired: 1 in, 2 out]
        n448 = property on="код" class="Str"("Visible"="Калибровка") -> ()  [unwired: 2 in, 2 out]
        n449 = Equal To 0?(x=w84) -> (x = 0?=w80:bool)
        n450 = Equal?(x=w84, y=u16 1) -> (x = y?=w81:bool)
        n451 = Not Equal?(x=w122, y=u32 9) -> (x != y?=w113:bool)
        n452 = String Subset(string=w125, length (rest)=2 ("length (rest)")) -> (substring=w120:string)  [unwired: 1 in]
        n453 = String Subset(string=w127, length (rest)=2 ("length (rest)")) -> (substring=w121:string)  [unwired: 1 in]
        n454 = And(x="Up Button", y="Down Button") -> (x .and. y?=w79:bool)
        n455 = property on="P_пластовое МПа" class="DigNum (strict)"("Visible"=w81) -> ()  [unwired: 2 in, 2 out]
        n456 = property on="Pпластовое" class="DigNum (strict)"("Visible"=w80) -> ()  [unwired: 2 in, 2 out]
        n457 = case shown="True" w79 {
          tunnel: "Up Button" -> [w161 _]
          tunnel: [w161 w162] -> w77
          tunnel: "Down Button" -> [w160 _]
          tunnel: [w160 w162] -> w75
          frame False {
          }
          frame True {
            w162 = FALSE
            n458 = local write "Down Button"(w162) -> ()
            n459 = local write "Up Button"(w162) -> ()
          }
        }
        n460 = Equal?(x=w121, y=w120) -> (x = y?=w115:bool)
        n461 = Equal?(x=w114, y=2) -> (x = y?=w118:bool)
        n462 = control-ref of="Клапана"() -> (w93:refnum<vi>)
        n463 = Or(x=w115, y=w118) -> (x .or. y?=w117:bool)
        n464 = Not(x=w113) -> (.not. x?=w116:bool)
        n465 = String Subset(string=w127, length (rest)=3 ("length (rest)")) -> (substring=w129:string)  [unwired: 1 in]
        n466 = And(x=w117, y=w116) -> (x .and. y?=w112:bool)
        n467 = call "Давление_код4_20.vi"("Уставка давления"="РД-1 1,0 МПА") -> ("mka"=w90:u16)  [unwired: 10 in]
        n468 = call "3_МПА.vi"("Уставка давления"="Регулятор\n давления") -> ("mka"=w141:u16)  [unwired: 10 in]
        n469 = Build Array(w141, w90, "клапан") -> (w143:u16[])
        n470 = control-ref of="РД-1 1,0 МПА"() -> (w88:refnum<vi>)
        n471 = case shown="True" w77 {
          tunnel: [w191 w200] -> w89
          tunnel: w88 -> [w191 w200]
          tunnel: "Мультипликатор" -> [_ w192]
          frame False {
          }
          frame True {
            n472 = local read "Р горное, МПа"() -> (w197:sgl)
            n473 = call-poly <vilib>:"PID.vi"("output range"=cluster{"output high":dbl, "output low":dbl} {"output high"=24000.0, "output low"=4000.0}, "dt (s)"="dt (s)", "PID gains"="PID gains", "process variable"=w197, "setpoint"=w192) -> ("output"=w198:dbl)  [unwired: 5 in, 1 out]
            "output" <- w198
            n474 = control-ref of="клапан"() -> (w194:refnum<vi>)
            n475 = To Word Integer(number=w198) -> (16bit integer=w195:i16)
            n476 = property class="DigNum (strict)"(reference=w194, "Value"=w195) -> ()  [unwired: 1 in, 2 out]
            n477 = property class="DigNum (strict)"(reference=w200, "Value"=0.0) -> ()  [unwired: 1 in, 2 out]
          }
        }
        n478 = case shown="True" w112 {
          tunnel: [w183 w190] -> w134
          tunnel: w129 -> [_ w189]
          tunnel: w127 -> [_ w188]
          tunnel: w111 -> [w183 _]
          tunnel: w110 -> [w182 w184]
          tunnel: [w181 w184] -> w109
          frame False {
            n479 = Increment(x=w182) -> (x+1=w181:i32)
          }
          frame True {
            n480 = Match Pattern(string=w188, regular expression=w189) -> (after substring=w186:string)  [unwired: 1 in, 3 out]
            n481 = String To Byte Array(string=w186) -> (unsigned byte array=w185:u8[])
            n482 = Type Cast(type=sgl 0.0, x=w185) -> (*(type *) &x=w190:sgl)
          }
        }
        "Ошибки" <- w109
        n483 = call "Read all.vi"("Овны"=w149, "3-регистра(501)"=w143, "Клапана"="Клапана", "error in (no error)"=w140) -> ("Овны 2"=w147:refnum<class "Modbus Master.lvclass">[], "Р пластовое"=→"P_пластовое МПа" →"P_пл.МПа":sgl, "Р горное"=w70:sgl, "Din"=w146:bool[], "Р атм."=→"Pатм. МПа" →"Атмосферное":sgl, "Температура"=→"Темп":sgl, "error out"=w148:errorcluster)  [unwired: 5 in]
        "Р горное, МПа" <- w70
        "P гор. МПа" <- w70
        n484 = Enqueue Element(queue=w153, element="stop 3", error in (no error)=w150) -> (queue out=w151:refnum<queue>, error out=w152:errorcluster)  [unwired: 1 in, 1 out]
        n485 = Index Array(array=w146) -> (element #1=→"Верхний":bool, element #2=w92:bool)  [unwired: 2 in]
        "Нижний" <- w92
        n486 = case shown="True" w75 {
          tunnel: w93 -> [_ w176]
          tunnel: w92 -> [_ w175]
          tunnel: w89 -> [_ w167]
          frame False {
          }
          frame True {
            n487 = control-ref of="Мультипликатор"() -> (w164:refnum<vi>)
            n488 = property class="Arr (strict)"(reference=w176) -> (reference out=w173:refnum<vi>, "Value"=w172:bool[])  [unwired: 1 in, 1 out]
            n489 = property class="Slide (strict)"(reference=w164) -> ("Value"=w163:dbl)  [unwired: 1 in, 2 out]
            n490 = call "Мульт_мпа.vi"("МПА"=w163) -> ("регулятор"=w165:dbl)  [unwired: 10 in]
            n491 = case shown="True" w175 {
              tunnel: [TRUE ("new element/subarray") FALSE] -> w170
              tunnel: w165 -> [w177 _]
              tunnel: [w177 0.0 ("регулятор")] -> w166
              frame False {
              }
              frame True {
              }
            }
            n492 = Replace Array Subset(array=w172, new element=w170, index=8) -> (w174:bool[])
            n493 = property class="Arr (strict)"(reference=w173, "Value"=w174) -> ()  [unwired: 1 in, 2 out]
            n494 = control-ref of="клапан"() -> (w169:refnum<vi>)
            n495 = property class="DigNum (strict)"(reference=w169, "Value"=i16 4000) -> ()  [unwired: 1 in, 2 out]
            n496 = property class="DigNum (strict)"(reference=w167, "Value"=w166) -> ()  [unwired: 1 in, 2 out]
          }
        }
        n497 = To Double Precision Float(number=w134) -> (double precision float=w73:dbl)
        "Рпласт." <- w73
        "Pпластовое" <- w73
        "Press" <- w73
        "P пл. МПа" <- w73
        n498 = Greater?(x=w70, y=sgl 70.0) -> (0:w68:bool)
        "x > y?" <- w68
        n499 = property on="x > y?" class="Bool (strict)"("Visible"=w68) -> ()  [unwired: 2 in, 2 out]
        n500 = Index Array(array="Клапана") -> (element #1=→"K1":bool, element #2=→"K2":bool, element #3=→"K3":bool, element #4=→"K4":bool, element #5=→"K5":bool, element #6=→"K6":bool, element #7=→"K7":bool, element #8=→"K8":bool, element #9=→"K9":bool, element #10=→"K10":bool, element #11=→"K11":bool)  [unwired: 12 in, 1 out]
        "Numeric 2" <- w114
      }
      n501 = case shown="True" TRUE {
        tunnel: [w62 errorcluster {"status"=FALSE, "code"=0, "source"=""} ("error IO")] -> w24
        tunnel: w25 -> [w62 w63]
        frame False {
        }
        frame True {
          n502 = Unbundle By Name(w63) -> ()  [unwired: 1 out]
        }
      }
      n503 = Release Queue(queue=w55, error in (no error)=w56) -> ()  [unwired: 1 in, 3 out]
      n504 = case shown="True" TRUE {
        tunnel: [w59 errorcluster {"status"=FALSE, "code"=0, "source"=""} ("error IO")] -> w21
        tunnel: w22 -> [w59 w60]
        frame False {
        }
        frame True {
          n505 = Unbundle By Name(w60) -> ()  [unwired: 1 out]
        }
      }
      n506 = for {
        tunnel: w54 -> [w66] mode=indexing
        tunnel: w24 -> [w67]
        n507 = call-dynamic "Shutdown.vi"("error in"=w67, "Modbus master in"=w66) -> ("error out"=w65:errorcluster)  [unwired: 9 in]
        n508 = Unbundle By Name(w65) -> ()  [unwired: 1 out]
      }
      n509 = VISA Close(VISA resource name=w38, error in (no error)=w21) -> ()  [unwired: 1 out]
    }
    frame Error {
      n510 = One Button Dialog(message="Проверте подключение к сети.", button name ("OK")="Выход") -> ()  [unwired: 1 out]
    }
  }
  n511 = case shown="True" TRUE {
    tunnel: [w1044 errorcluster {"status"=FALSE, "code"=0, "source"=""} ("error IO")] -> w2
    tunnel: w3 -> [w1044 w1045]
    frame False {
    }
    frame True {
      n512 = Unbundle By Name(w1045) -> ()  [unwired: 1 out]
    }
  }
  n513 = control-ref of="This Application"() -> (w8:refnum<vi>)
  n514 = property class="App"(reference=w8, error in=w2) -> ("App.Kind"=w9:T10)  [unwired: 2 out]
  n515 = case shown="\"Run Time System\"" w9 {
    frame "invalid app kind", Default {
    }
    frame "Development System" {
    }
    frame "Run Time System" {
      n516 = Quit LabVIEW(quit? (T)=TRUE) -> ()
    }
  }
